vi "MAIN_DSOM.vi"(6 "Y-Max / [V]":dbl=9.0 min=0.0 max=10.0, 7 "X-Max / [V]":dbl=9.0 min=0.0 max=10.0, 8 "Y-Pixels":u32=10 min=2, 9 "Y-Min / [V]":dbl=1.0 min=0.0 max=10.0, 10 "X-Min / [V]":dbl=1.0 min=0.0 max=10.0, 11 "X-Pixels":u32=10 min=2 max=4000) -> ()   [LabVIEW 2009]
uses:
  <vilib>/DAQmx/create/channels.llb/DAQmx Create Channel (DO-Digital Output).vi
  <vilib>/DAQmx/configure/timing.llb/DAQmx Timing (Sample Clock).vi
  <vilib>/DAQmx/write.llb/DAQmx Write (Analog 2D DBL NChan NSamp).vi
  <vilib>/DAQmx/write.llb/DAQmx Write (Digital 1D U8 1Chan NSamp).vi
  Program Files/National Instruments/LabVIEW 2009/resource/objmgr/daqmx.rc
  <vilib>/DAQmx/create/channels.llb/DAQmx Create Channel (AO-Voltage-Basic).vi
  atmcd32d.llb/Shutter_mode typedef.ctl
  atmcd32d.llb/Shutter_type typedef.ctl
  atmcd32d.llb/AcquisitionMode_mode typedef.ctl
  atmcd32d.llb/ReadMode_mode typedef.ctl
  atmcd32d.llb/TriggerMode_mode typedef.ctl
  <vilib>/DAQmx/create/channels.llb/DAQmx Create Channel (CO-Pulse Generation-Frequency).vi
  <vilib>/DAQmx/configure/timing.llb/DAQmx Timing (Implicit).vi
  atmcd32d.llb/EMGainMode_mode typedef.ctl
panel:
  in  "Average or max.\nIntensity":bool
  in  "Scanner Divider":i32=2
  in  "Learning loop":bool=TRUE
  in  "Normalize\nPicture Image":bool=TRUE
  in  "SCANNER EMERGENCY":bool
  out "Cursor Y":i16
  out "Cursor X":i16
  out "Waveform Chart 2":dbl(graph)
  in  "Measurement Mode":enum32{"Picture", "Line", "Point"}(tab)
  out "?":bool
  out "Slide":i32
  out "Programming scanner":u8(slide) caption="Accquire Picture" scale=0.0..100.0
  in  "?":enum32{"Picture", "ROI", "3D-Stack"}(tab)
  in  "Overview":bool
  out "?":bool
  in  "Square":bool
  in  "x-Pixel":u16=100
  in  "y-Pixel":u16=100
  in  "Picture size":dbl=20.0 min=0.1 max=200.0 format="%1.1f um"
  in  "?":dbl=20.0 min=0.1 max=200.0 format="%1.1f um"
  in  "z-Position":dbl=50.0 min=0.0 max=200.0 format="%1.3f um"
  in  "y-Position":dbl=50.0 min=0.0 max=200.0 format="%1.3f um"
  in  "x-Position":dbl=50.0 min=0.0 max=200.0 format="%1.3f um"
  in  "Accquire":bool
  out "?":bool
  in  "lower limit":i32=10 min=0
  in  "x-Pixel":i32=10 min=0
  in  "Square":bool
  in  "y-Pixel":i32=10 min=0
  in  "ROI":bool
  in  "left limit":i32=10 min=0
  out "?":bool
  in  "Zoom":bool
  out "?":bool
  in  "lower left":bool
  in  "upper right":bool
  in  "Step-width [nm]":i32
  in  "Slides":i32
  in  "Stack?":bool
  out "y":dbl format="%.1f nm"
  out "x":dbl format="%.1f nm"
  in  "?":enum32{"Stage", "Mirror"}(radio)
  in  "?":enum32{"Confocal", "High Res"}(radio)=enum."High Res"
  in  "?":enum32{"x-y", "x-z", "y-z"}(radio)
  out "Measurement time / [s]":u32
  in  "Save":bool
  in  "?":enum32{"Stage", "Mirror"}(radio)
  in  "Start Point":dbl
  in  "?":enum32{"Confocal", "High Res"}(radio)
  out "?":bool
  in  "Accquire":bool
  in  "z-Position":dbl=50.0 min=0.0 max=200.0 format="%1.3f um"
  in  "y-Position":dbl=50.0 min=0.0 max=200.0 format="%1.3f um"
  in  "x-Position":dbl=50.0 min=0.0 max=200.0 format="%1.3f um"
  in  "?":enum32{"Picture", "Int Trace", "Video"}(radio)
  in  "?":enum32{"Stage", "Mirror"}(radio)
  in  "Save":bool
  in  "Num of Pictures":i32=3
  out "?":dbl format="%1.3f um"
  out "?":dbl format="%1.3f um"
  out "Intensity Graph":i32[][](graph)
  out "Wavelength_Percent":i32[](array[numeric])
  out "Picture Time":dbl
  out "Exposure Time":u32[][](array[numeric])
  out "Power settings":dbl[][](array[numeric])
  out "Pulse per Wavelength":u8[](array[numeric])
  out "Wavelength":i32[](array[numeric])
  in  "?":T1(tab)=enum."Andor IXon 860"
  in  "Measurement Type":enum32{"Point", "Line", "Area", "Cube"}(ring)
  out "?":bool
  in  "Seed Laser Power 2":i8(knob) min=0 max=100 scale=0.0..100.0
  in  "Laser 2":bool caption="Seed Laser"
  out "?":bool
  in  "PicoQuant Laser Head":bool
  out "Time per Pixel / [ms]":dbl format="%#_6f"
  in  "stop":bool
  in  "Start":bool
  out "Total scanning time / [s]":dbl
  out "Running":bool
  in  "Laser Power Type":T2(ring)
  out "Pictures per pixel":u8
  in  "Number of active Koheras lines":i8=1 min=1 max=8
  out "Actual Power Level / [%]":i8(knob) scale=0.0..100.0
  out "active 1":bool
  out "active 8":bool
  out "active 7":bool
  out "active 6":bool
  out "active 5":bool
  out "active 4":bool
  out "active 3":bool
  out "active 2":bool
  in  "?":T2(tab)
  in  "Number of active Koheras lines":i8=1 min=1 max=8
  out "Command":string
  out "Programming AOTF":bool
  in  "Set Manual":bool
  in  "Exposure\nTime / [us]":u32=100 min=1
  in  "Line 1":i32(slide) min=0 max=100 scale=0.0..100.0
  in  "Line 1":i32(slide)=470 min=470 max=730 scale=470.0..730.0
  in  "Line 2":i32(slide)=470 min=470 max=730 scale=470.0..730.0
  in  "Line 3":i32(slide)=470 min=470 max=730 scale=470.0..730.0
  in  "Line 4":i32(slide)=470 min=470 max=730 scale=470.0..730.0
  in  "Line 5":i32(slide)=470 min=470 max=730 scale=470.0..730.0
  in  "Line 6":i32(slide)=470 min=470 max=730 scale=470.0..730.0
  in  "Line 7":i32(slide)=470 min=470 max=730 scale=470.0..730.0
  in  "Line 8":i32(slide)=470 min=470 max=730 scale=470.0..730.0
  in  "Line 2":i32(slide) min=0 max=100 scale=0.0..100.0
  in  "Line 3":i32(slide) min=0 max=100 scale=0.0..100.0
  in  "Line 4":i32(slide) min=0 max=100 scale=0.0..100.0
  in  "Line 5":i32(slide) min=0 max=100 scale=0.0..100.0
  in  "Line 6":i32(slide) min=0 max=100 scale=0.0..100.0
  in  "Line 7":i32(slide) min=0 max=100 scale=0.0..100.0
  in  "Line 8":i32(slide) min=0 max=100 scale=0.0..100.0
  in  "Exposure\nTime / [us]":u32=100 min=1
  in  "Exposure\nTime / [us]":u32=100 min=1
  in  "Exposure\nTime / [us]":u32=100 min=1
  in  "Exposure\nTime / [us]":u32=100 min=1
  in  "Exposure\nTime / [us]":u32=100 min=1
  in  "Exposure\nTime / [us]":u32=100 min=1
  in  "Exposure\nTime / [us]":u32=100 min=1
  in  "Exposure\nTime 9 / [us]":u32=100 min=1
  in  "Exposure Time\n/ [us]":i32[](array[numeric]) min=1 max=1000000
  in  "Exposure Time\n/ [us]":i32[](array[numeric]) min=1 max=1000000
  in  "Exposure Time\n/ [us]":i32[](array[numeric]) min=1 max=1000000
  in  "Exposure Time\n/ [us]":i32[](array[numeric]) min=1 max=1000000
  in  "Exposure Time\n/ [us]":i32[](array[numeric]) min=1 max=1000000
  in  "Exposure Time\n/ [us]":i32[](array[numeric]) min=1 max=1000000
  in  "Exposure Time\n/ [us]":i32[](array[numeric]) min=1 max=1000000
  in  "Exposure Time\n/ [us]":i32[](array[numeric]) min=1 max=1000000
  in  "Used Power\nEntries":u8=1 min=1
  in  "Power":dbl[](array[numeric]) min=0.0 max=100.0
  in  "Used Power\nEntries":u8=1 min=1
  in  "Power":dbl[](array[numeric]) min=0.0 max=100.0
  in  "Used Power\nEntries":u8=1 min=1
  in  "Power":dbl[](array[numeric]) min=0.0 max=100.0
  in  "Used Power\nEntries":u8=1 min=1
  in  "Power":dbl[](array[numeric]) min=0.0 max=100.0
  in  "Used Power\nEntries":u8=1 min=1
  in  "Power":dbl[](array[numeric]) min=0.0 max=100.0
  in  "Used Power\nEntries":u8=1 min=1
  in  "Power":dbl[](array[numeric]) min=0.0 max=100.0
  in  "Used Power\nEntries":u8=1 min=1
  in  "Power":dbl[](array[numeric]) min=0.0 max=100.0
  in  "Used Power\nEntries":u8=1 min=1
  in  "Line 1":i32(slide)=470 min=470 max=730 scale=470.0..730.0
  in  "Line 2":i32(slide)=470 min=470 max=730 scale=470.0..730.0
  in  "Line 3":i32(slide)=470 min=470 max=730 scale=470.0..730.0
  in  "Line 4":i32(slide)=470 min=470 max=730 scale=470.0..730.0
  in  "Line 5":i32(slide)=470 min=470 max=730 scale=470.0..730.0
  in  "Line 6":i32(slide)=470 min=470 max=730 scale=470.0..730.0
  in  "Line 7":i32(slide)=470 min=470 max=730 scale=470.0..730.0
  in  "Line 8":i32(slide)=470 min=470 max=730 scale=470.0..730.0
  in  "Power":dbl[](array[numeric]) min=0.0 max=100.0
  in  "Proportional\nto Intensity 8":bool caption="Proportional\nto Intensity"
  in  "Exposure\nTime / [us]":u32=100 min=1
  in  "Proportional\nto Intensity 7":bool caption="Proportional\nto Intensity"
  in  "Exposure\nTime / [us]":u32=100 min=1
  in  "Proportional\nto Intensity 6":bool caption="Proportional\nto Intensity"
  in  "Exposure\nTime / [us]":u32=100 min=1
  in  "Proportional\nto Intensity 5":bool caption="Proportional\nto Intensity"
  in  "Exposure\nTime / [us]":u32=100 min=1
  in  "Proportional\nto Intensity 4":bool caption="Proportional\nto Intensity"
  in  "Exposure\nTime / [us]":u32=100 min=1
  in  "Proportional\nto Intensity 3":bool caption="Proportional\nto Intensity"
  in  "Exposure\nTime / [us]":u32=100 min=1
  in  "Proportional\nto Intensity 2":bool caption="Proportional\nto Intensity"
  in  "Exposure\nTime / [us]":u32=100 min=1
  in  "Proportional\nto Intensity":bool
  in  "Steps":u8=2 min=2
  in  "Last Intensity":i8=100 min=0 max=100
  in  "First Intensity":i8=1 min=1 max=100
  in  "Steps":u8=2 min=2
  in  "Last Intensity":i8=100 min=0 max=100
  in  "First Intensity":i8=1 min=1 max=100
  in  "Steps":u8=2 min=2
  in  "Last Intensity":i8=100 min=0 max=100
  in  "First Intensity":i8=1 min=1 max=100
  in  "Steps":u8=2 min=2
  in  "Last Intensity":i8=100 min=0 max=100
  in  "First Intensity":i8=1 min=1 max=100
  in  "Steps":u8=2 min=2
  in  "Last Intensity":i8=100 min=0 max=100
  in  "First Intensity":i8=1 min=1 max=100
  in  "Steps":u8=2 min=2
  in  "Last Intensity":i8=100 min=0 max=100
  in  "First Intensity":i8=1 min=1 max=100
  in  "Steps":u8=2 min=2
  in  "Last Intensity":i8=100 min=0 max=100
  in  "First Intensity":i8=1 min=1 max=100
  in  "Steps":u8=2 min=2
  in  "Last Intensity":i8=100 min=0 max=100
  in  "First Intensity":i8=1 min=1 max=100
  in  "Line 1":i32(slide)=470 min=470 max=730 scale=470.0..730.0
  in  "Line 2":i32(slide)=470 min=470 max=730 scale=470.0..730.0
  in  "Line 3":i32(slide)=470 min=470 max=730 scale=470.0..730.0
  in  "Line 4":i32(slide)=470 min=470 max=730 scale=470.0..730.0
  in  "Line 5":i32(slide)=470 min=470 max=730 scale=470.0..730.0
  in  "Line 6":i32(slide)=470 min=470 max=730 scale=470.0..730.0
  in  "Line 7":i32(slide)=470 min=470 max=730 scale=470.0..730.0
  in  "Line 8":i32(slide)=470 min=470 max=730 scale=470.0..730.0
  in  "Exposure\nTime / [us]":u32=100 min=1
  out "active 9":bool
  out "Interlock":bool
  out "Reset Interlock":bool
  out "?":bool
  in  "Seed Laser Power":i8(knob) min=0 max=100 scale=0.0..100.0
  in  "Laser":bool caption="Seed Laser"
  out "Actual Power Level / [%]":i8(knob) scale=0.0..100.0
  out "Output Photodiode current":i32(graph)
  out "Diode current":cluster{i32, i32, i32}(graph)
  out "Temperature Case":string
  out "Temperature Booster":string
  out "Temperature Preamplifier":string
  out "Temperature Seed Laser":string
  out "SuperK Firmware rev. Hardware":string
  out "SuperK Firmware rev. Display":string
  out "SuperK Firmware rev. Main":string
  out "SuperK Serial No.":string
  out "Board Version":string
  out "Board Serial":string
  out "Board ID":string
  in  "Y-Voltage":dbl=5.0 min=0.0 max=10.0 format="%.6g"
  in  "X-Voltage":dbl=5.0 min=0.0 max=10.0 format="%.6g"
  in  "Set Manual":bool
  in  "Choose Position":dbl min=-10.0 max=10.0 format="%.6g"
  out "Numeric":dbl
  out "Fixed Position / [mm]":dbl format="%.6g"
  in  "Reset Fix Position":bool
  in  "Fix Position":bool
  in  "Move Down":bool
  in  "Move Up":bool
  out "Moving Speed / [%]":i8(knob) scale=0.0..100.0
  in  "Clutch":bool
  out "Actual Microscope Position / [mm]":dbl format="%.6f"
  in  "Numeric 2":i32=10
  out "Differenz":dbl format="%.6f"
  out "actual scan stage position":dbl[](array[numeric]) format="%.6f"
  in  "Shut down\ncamera":bool
  in  "Exposure time / ms":i32=1 min=1 max=5000
  in  "y-pixels":u32=1 min=1 max=1024
  in  "x-pixels":u32=1 min=1 max=1024
  in  "target temperature / [°C]":i32(knob)=40 min=0 max=70 scale=0.0..70.0 scale format="-%.0f"
  out "Temp-stabilized":bool
  out "On/Off":bool
  out "act. temperature / [°C]":dbl
  in  "Cooling":bool
  out "Y-Pixels":dbl
  out "X-Pixels":dbl
  in  "Zoom":bool
  in  "upper right 2":bool
  in  "lower left 2":bool
  in  "x- lower left":u8 max=128
  in  "x- upper right":u8=128 max=128
  in  "y- lower left":u8 max=128
  in  "y-upper right":u8=128 max=128
  in  "gain":i32
  in  "mode":T3
  out "sigx":dbl
  out "sigy":dbl
  out "Signalverlaufsdiagramm":cluster{dbl, dbl}(graph)
  in  "Main Start Clock out":tag="/Dev3/PFI36"
  in  "Analog-Channel Y":tag="Dev1/ao1"
  in  "Analog-Channel X":tag="Dev1/ao0"
  in  "Heidenhain_Seriell":refnum<visa-resource-name>="COM4"
  in  "AOTF Line 1":tag="Dev2/ao0"
  in  "AOTF Line 2":tag="Dev2/ao1"
  in  "AOTF Line 3":tag="Dev2/ao2"
  in  "AOTF Line 4":tag="Dev2/ao3"
  in  "AOTF Line 5":tag="Dev2/ao4"
  in  "AOTF Line 6":tag="Dev2/ao5"
  in  "AOTF Line 7":tag="Dev2/ao6"
  in  "AOTF Line 8":tag="Dev2/ao7"
  in  "Delayed  Main Start Clock in":tag="/Dev3/PFI28"
  in  "AOTF-Digital out":tag="Dev2/port0"
  in  "AOTF-Analog Min Voltage / [V]":dbl
  in  "AOTF-Analog Max Voltage / [V]":dbl=10.0
  in  "Delay / [us]":i32=10 min=1
  in  "Delayed Startclock out":tag="Dev3/ctr1" caption="Delayed Start Clock Out"
  in  "Main Startclock In":tag="/Dev3/PFI0" caption="Main Startclock in"
  in  "20 MHz-Clock":tag="/Dev3/20MHzTimebase" caption="20MHz-Clock for \nDelay-Counting"
  in  "Sample-Clock Out":tag="/Dev1/ao/SampleClock"
  in  "Power Driver":tag="Dev1/port2"
  in  "Clock out":tag="Dev3/ctr7"
  in  "Koheras-AOTF-Controller":refnum<visa-resource-name>="USB0::0x16C7::0x0001::NI-VISA-10001::RAW"
  in  "Koheras Seed Laser":refnum<visa-resource-name>="COM5"
  in  "Picture Clock out":tag="Dev3/ctr3" caption="Pixel Clock out"
  in  "AOTF-Digital switch in":tag="/Dev2/PFI0"
  in  "AOTF-Analog switch in":tag="/Dev2/PFI0"
  in  "Picture Clock Main out":tag="Dev3/ctr5"
  in  "Picture Start Clock in":tag="/Dev3/PFI20"
  in  "Blanking Out":tag="Dev1/port0"
  in  "Picture Clock Main in":tag="/Dev3/PFI12"
  in  "PI E710":u16(ring) items=["COM1", "COM2", "COM3", "COM4", "COM5", "COM6", "COM7", "COM8", "COM9"]
  # "lower left corner"
  # "from cursor"
  # "Pixelsize"
  # "Scan-\ntype"
  # "Laser Power Settings"
  # "Wavelength"
  # "Power"
  # "Koheras-AOTF"
  # "PicoQuant"
  # "Wavelength"
  # "PicoQuant"
  # "Koheras-AOTF"
  # "Wavelength"
  # "In case of proportional exposure to intensity setting, setted exposure time counts for 100% intensity"
  # "PicoQuant"
  # "Koheras-AOTF"
  # "Interlock"
  # "Laser Power Settings"
  # "Temperature"
  # "Koheras\nHardware Version"
  # "Koheras AOTF"
  # "Manual Positioning"
  # "PI  E710-Scanner"
  # "x"
  # "y"
  # "z"
  # "Camera binning"
  # "X"
  # "Camera cooling"
  # "Camera read out"
  # "Scanner"
  # "Timing"
  # "Camera"
  # "AOTF-Analog"
  # "AOTF-Digital"
  # "Mikroskope z-Position"
  # "Position Controller"
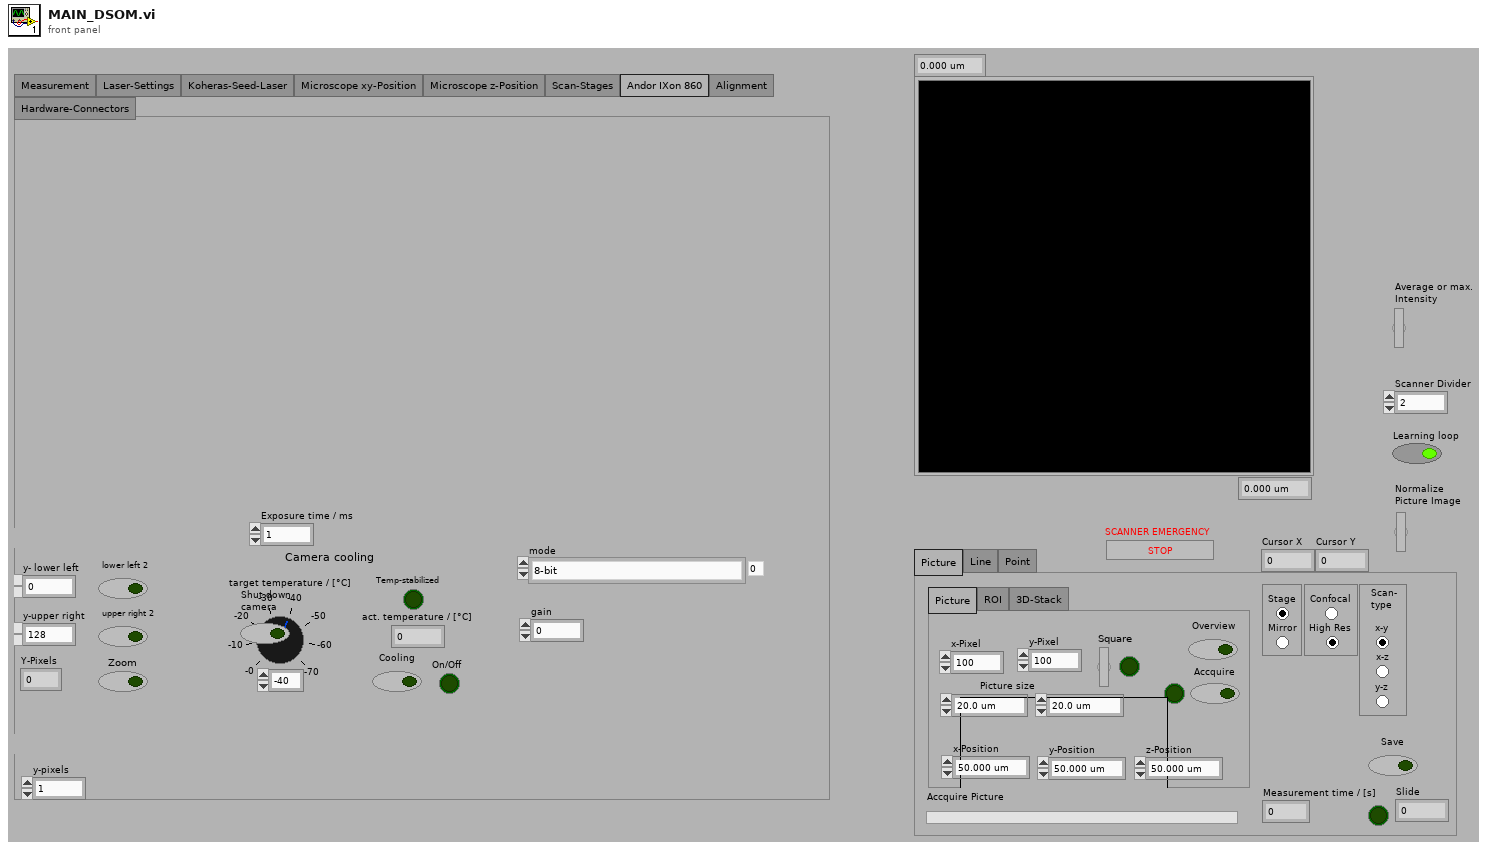
[diagram p1: front panel]
types:
  T1 = enum32{"Measurement", "Laser-Settings", "Koheras-Seed-Laser", "Microscope xy-Position", "Microscope z-Position", "Scan-Stages", "Andor IXon 860", "Alignment", "Hardware-Connectors"}
  T2 = enum32{"Static Power", "Dynamic Power Discrete", "Dynamic Power Ramp"}
  T3 = typedef "EMGainMode_mode typedef.ctl" = enum16{"8-bit", "12-bit", "Linear", "Real"}
  T4 = cluster{string, "cancelled":bool, "error out":errorcluster, bool, "Slides":i32, string}
  T5 = cluster{"Value":i8, "Value":i32[], "Value":i32[], "Set Manual":bool}
  T6 = cluster{"x-Pixel":u16, "y-Pixel":u16, "x-Position":dbl, "y-Position":dbl, "Picture size":dbl, dbl, enum32{"x-y", "x-z", "y-z"}, "z-Position":dbl}
  T7 = typedef "Shutter_mode typedef.ctl" = enum16{"Auto", "Open", "Close"}
  T8 = typedef "Shutter_type typedef.ctl" = enum16{"TTL Low", "TTL High"}
  T9 = typedef "TriggerMode_mode typedef.ctl" = enum16{"Internal", "External", "N/A (2)", "N/A (3)", "N/A (4)", "N/A (5)", "External Start"}
  T10 = typedef "ReadMode_mode typedef.ctl" = enum16{"Full Vertical Binning", "Multi-Track", "Random-Track", "Single-Track", "Image"}
  T11 = typedef "AcquisitionMode_mode typedef.ctl" = enum16{"Reserved (0)", "Single Scan", "Accumulate", "Kinetics", "Fast Kinetics", "Run Till Abort", "Reserved (6)", "Reserved (7)", "Reserved (8)", "Time Delayed Integration"}
  T12 = cluster{"dimension size":i32, "dimension size":i32, "dimension size":i32, "dimension size":i32}
  T13 = cluster{"Acquis. mode":T11, "Read mode":T10, "Horizontal bin":i32, "Vertical bin":i32, "x-min":i32, "x-max":i32, "y-min":i32, "y-max":i32, "Trigger mode":T9, " Exposure time":sgl, "AD channel":i32, "Num of Pictures":i32, "Shutter type":T8, "Shutter mode":T7, "Shutter\nopeningtime":i32, "Shutter\nclosingtime":i32}
  T14 = cluster{cluster{"dimension size":i32, "dimension size":i32, "dimension size":i32, "dimension size":i32}, i32[], "Picture Data":dbl[][], u32[], "millisecond timer value":u32, dbl[][], i32[][], cluster{"Acquis. mode":T11, "Read mode":T10, "Horizontal bin":i32, "Vertical bin":i32, "x-min":i32, "x-max":i32, "y-min":i32, "y-max":i32, "Trigger mode":T9, " Exposure time":sgl, "AD channel":i32, "Num of Pictures":i32, "Shutter type":T8, "Shutter mode":T7, "Shutter\nopeningtime":i32, "Shutter\nclosingtime":i32}, "Boolean array":bool[], cluster{dbl[], dbl[]}, "cluster":cluster{"x-Pixel":u16, "y-Pixel":u16, "x-Position":dbl, "y-Position":dbl, "Picture size":dbl, dbl, enum32{"x-y", "x-z", "y-z"}, "z-Position":dbl}}
  T15 = cluster{"Boolean array[0]":bool, "Boolean array[1]":bool, "Boolean array[2]":bool, "Boolean array[3]":bool, "Boolean array[4]":bool, "Boolean array[5]":bool, "Boolean array[6]":bool, "Boolean array[7]":bool, "Boolean array[8]":bool}
  T16 = cluster{dbl, "X-Pixels":u32, "Y-Pixels":u32, "X-Min / [V]":dbl, "X-Max / [V]":dbl, "Y-Min / [V]":dbl, "Y-Max / [V]":dbl}
  T17 = cluster{"AOTF Line 1":tag, "AOTF Line 2":tag, "AOTF Line 3":tag, "AOTF Line 4":tag, "AOTF Line 5":tag, "AOTF Line 6":tag, "AOTF Line 7":tag, "AOTF Line 8":tag}
  T18 = cluster{"Main Start Clock out":tag, "Analog-Channel X":tag, "Analog-Channel Y":tag, "Sample-Clock Out":tag}
  T19 = cluster{"AOTF-Digital switch in":tag, "Picture Clock out":tag, "AOTF-Analog switch in":tag, "Picture Clock Main out":tag, "Picture Start Clock in":tag, "Picture Clock Main in":tag, "Blanking Out":tag, "Delayed  Main Start Clock in":tag, "AOTF-Digital out":tag}
  T20 = cluster{"Delay / [us]":i32, "Delayed Startclock out":tag, "Main Startclock In":tag, "20 MHz-Clock":tag}
  T21 = cluster{"Value":bool, "Value":bool[], "Value":bool[], "Set Manual":bool}
  T22 = cluster{"Cursor.Cursor X":dbl, "Cursor.Cursor Y":dbl}
  T23 = cluster{"x- lower left":u8, "y- lower left":u8, "x- upper right":u8, "y-upper right":u8}
  T24 = cluster{cluster{"x- lower left":u8, "y- lower left":u8, "x- upper right":u8, "y-upper right":u8}, cluster{"dimension size":i32, "dimension size":i32, "dimension size":i32, "dimension size":i32}, "lower left 2":bool, "upper right 2":bool}
  T25 = cluster{"left limit":i32, "lower limit":i32, "x-Pixel":i32, "y-Pixel":i32}
  T26 = cluster{"left limit":i32, i32, "lower limit":i32, i32}
  T27 = typedef "Error Code Enum typedef.ctl" = enum32{"N/A (0)", "DRV_ERROR_CODES", "DRV_SUCCESS", "DRV_VXDNOTINSTALLED", "DRV_ERROR_SCAN", "DRV_ERROR_CHECK_SUM", "DRV_ERROR_FILELOAD", "DRV_UNKNOWN_FUNC", "DRV_ERROR_VXD_INIT", "DRV_ERROR_ADDRESS", "DRV_ERROR_PAGELOCK", "DRV_ERROR_PAGEUNLOCK", "DRV_ERROR_BOARDTEST", "DRV_ERROR_ACK", "DRV_ERROR_UP_FIFO", "DRV_ERROR_PATTERN", "N/A (16)", "DRV_ACQUISITION_ERRORS", "DRV_ACQ_BUFFER", "DRV_ACQ_DOWNFIFO_FULL", "DRV_PROC_UNKONWN_INSTRUCTION", "DRV_ILLEGAL_OP_CODE", "DRV_KINETIC_TIME_NOT_MET", "DRV_ACCUM_TIME_NOT_MET", "DRV_NO_NEW_DATA", "N/A (25)", "DRV_SPOOLERROR", "N/A (27)", "N/A (28)", "N/A (29)", "N/A (30)", "N/A (31)", "N/A (32)", "DRV_TEMPERATURE_CODES", "DRV_TEMPERATURE_OFF", "DRV_TEMPERATURE_NOT_STABILIZED", "DRV_TEMPERATURE_STABILIZED", "DRV_TEMPERATURE_NOT_REACHED", "DRV_TEMPERATURE_OUT_RANGE", "DRV_TEMPERATURE_NOT_SUPPORTED", "DRV_TEMPERATURE_DRIFT", "N/A (41)", "N/A (42)", "N/A (43)", "N/A (44)", "N/A (45)", "N/A (46)", "N/A (47)", "N/A (48)", "DRV_GENERAL_ERRORS", "DRV_INVALID_AUX", "DRV_COF_NOTLOADED", "DRV_FPGAPROG", "DRV_FLEXERROR", "DRV_GPIBERROR", "N/A (55)", "N/A (56)", "N/A (57)", "N/A (58)", "N/A (59)", "N/A (60)", "N/A (61)", "N/A (62)", "N/A (63)", "DRV_DATATYPE", "DRV_DRIVER_ERRORS", "DRV_P1INVALID", "DRV_P2INVALID", "DRV_P3INVALID", "DRV_P4INVALID", "DRV_INIERROR", "DRV_COFERROR", "DRV_ACQUIRING", "DRV_IDLE", "DRV_TEMPCYCLE", "DRV_NOT_INITIALIZED", "DRV_P5INVALID", "DRV_P6INVALID", "DRV_INVALID_MODE", "DRV_INVALID_FILTER", "DRV_I2CERRORS", "DRV_I2CDEVNOTFOUND", "DRV_I2CTIMEOUT", "DRV_P7INVALID", "N/A (84)", "N/A (85)", "N/A (86)", "N/A (87)", "N/A (88)", "N/A (89)", "DRV_IOCERROR", "DRV_VRMVERSIONERROR"}
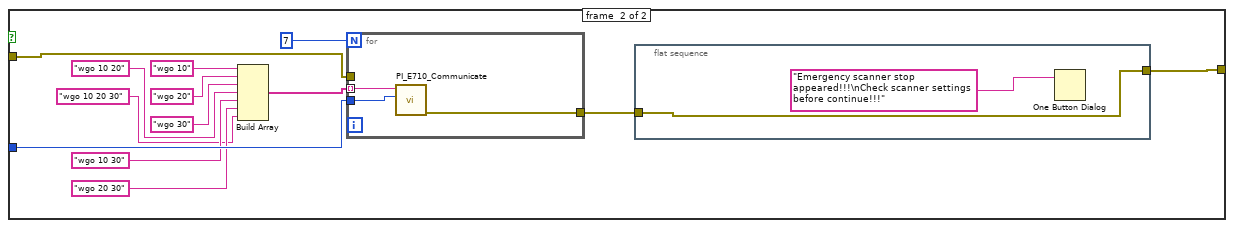
[diagram p2: hidden frame]
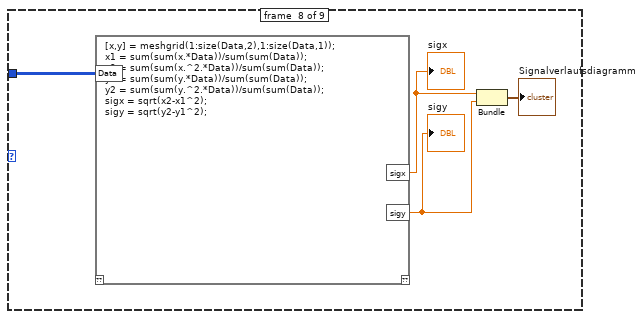
[diagram p9: hidden frame]
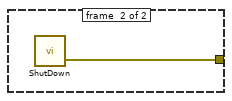
[diagram p11: hidden frame]
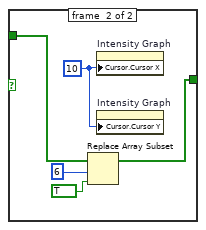
[diagram p12: hidden frame]
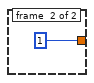
[diagram p13: hidden frame]
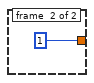
[diagram p14: hidden frame]
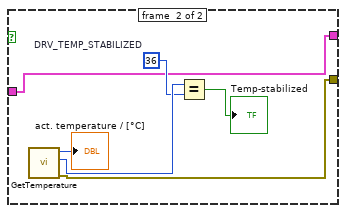
[diagram p15: hidden frame]
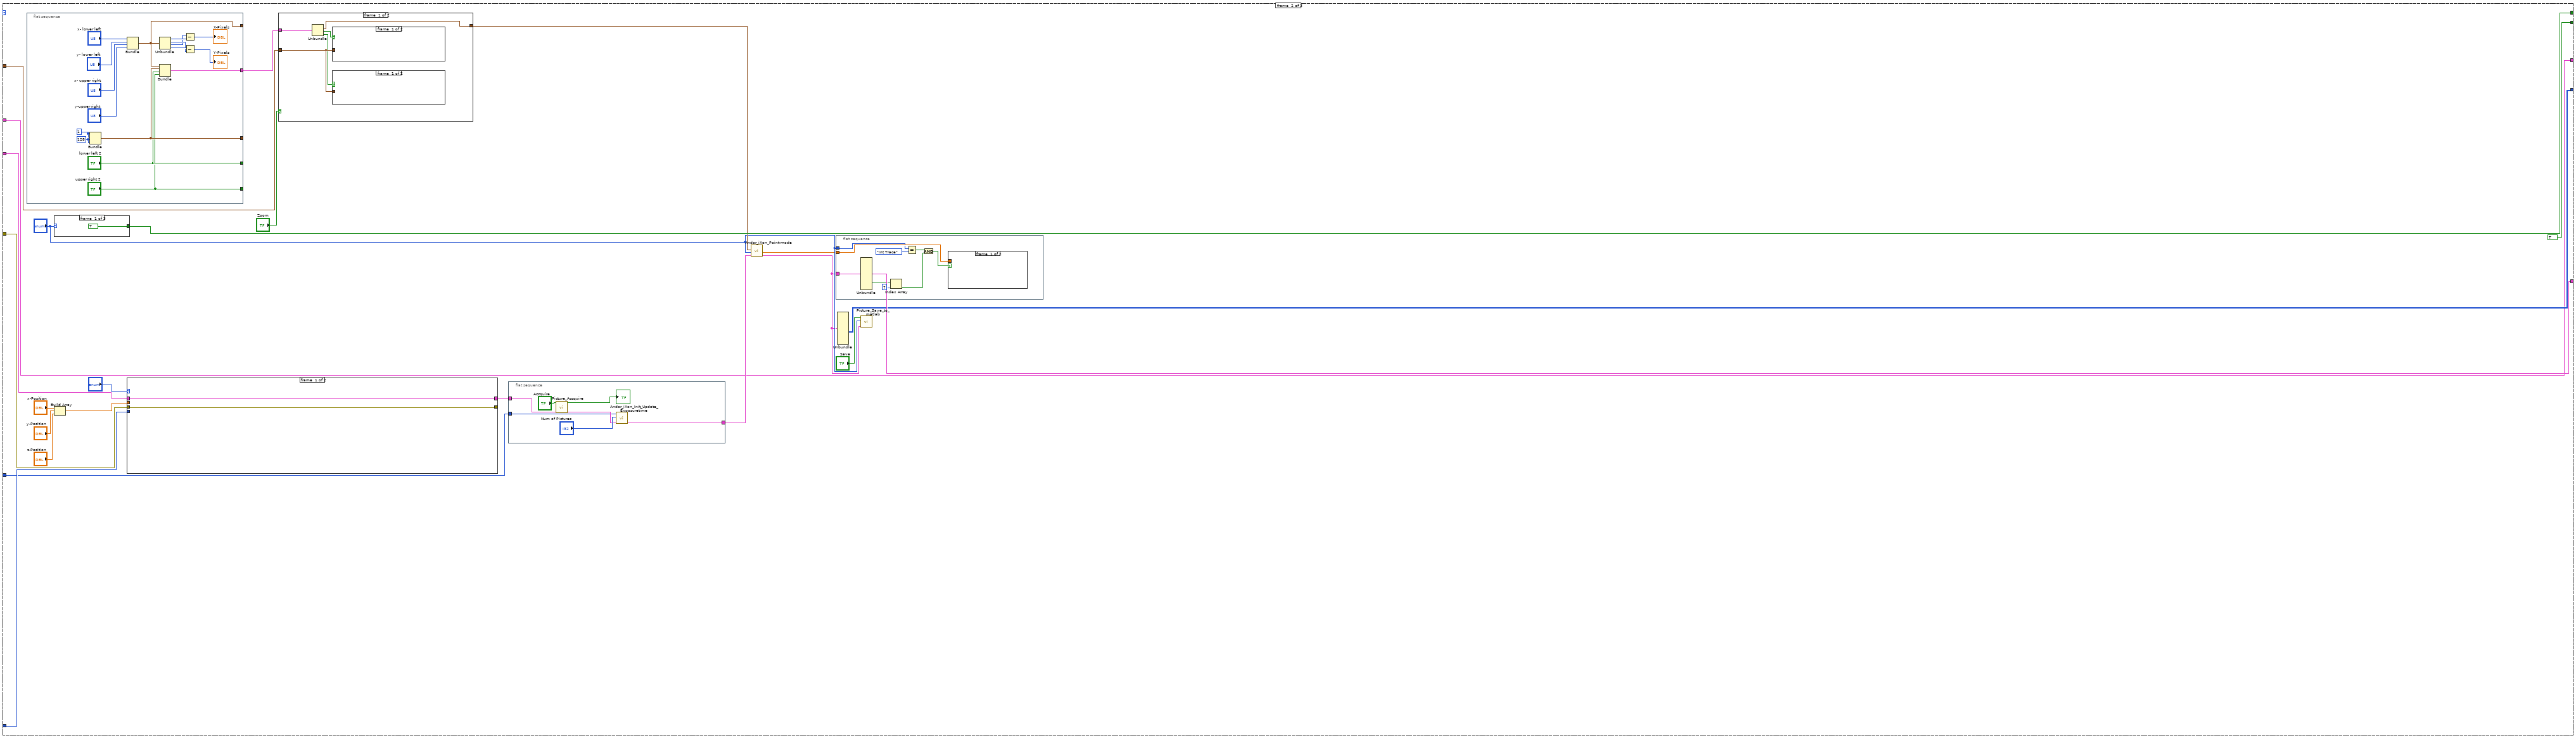
[diagram p17: hidden frame]
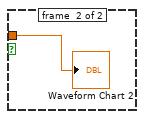
[diagram p18: hidden frame]
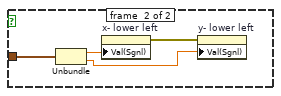
[diagram p19: hidden frame]
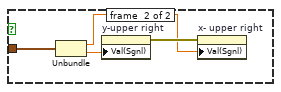
[diagram p20: hidden frame]
diagram:
  w3 = 1  # System no.
  w18 = 10214 items=["High"=10192, "Low"=10214] ("Idle State 2")
  w8 = bool[] [FALSE, FALSE, FALSE, FALSE, FALSE, FALSE, FALSE, FALSE] ("appended array")
  w19 = 10123 items=["Finite Samples"=10178, "Continuous Samples"=10123] ("sample mode")
  w28 = 1 items=["one channel for each line", "one channel for all lines"] ("line grouping")
  n1 = flat-sequence {
    tunnel: [w72] -> w2
    frame #0 {
      w48 = 0.0 ("element")
      w60 = 3  # Num of Pictures
      w51 = 128  # y-max
      w52 = 128  # y-min
      w53 = 1  # x-max
      w54 = 1  # x-min
      w64 = 1  # Vertical bin
      w65 = 1  # Horizontal bin
      w56 = 0  # Shutter closingtime
      w57 = 0  # Shutter openingtime
      w58 = Shutter_mode_typedef."Auto"  # Shutter mode
      w59 = Shutter_type_typedef."TTL Low"  # Shutter type
      w61 = 0  # AD channel
      w62 = sgl 0.05  # Exposure time
      w63 = TriggerMode_mode_typedef."Internal"  # Trigger mode
      w66 = ReadMode_mode_typedef."Image"  # Read mode
      w67 = AcquisitionMode_mode_typedef."Kinetics"  # Acquis. mode
      w76 = 128 ("dimension size")
      w77 = 1 ("dimension size")
      w73 = dbl[][] []  # Picture Data
      w91 = 1  # element
      n2 = Build Array "Scanner 1 Range"(0.0 ("y"), 200.0 ("y")) -> (w83:dbl[])
      n3 = Build Array "Scanner 2 Range"(0.0 ("y"), 200.0 ("y")) -> (w82:dbl[])
      n4 = Build Array "Scanner 3 Range"(0.0 ("element"), 200.0 ("y")) -> (w81:dbl[])
      n5 = Initialize Array "Pixels_Confocal"(w91, 512 ("dimension size"), 512 ("dimension size")) -> (w68:i32[][])
      n6 = Build Array "Scanner position"(w48, w48, w48) -> (w46:dbl[])
      n7 = Bundle("dimension size"=w77, "dimension size"=w77, "dimension size"=w76, "dimension size"=w76) -> (w75:T12)  [unwired: 1 out]
      n8 = Initialize Array(0, 16384 ("dimension size")) -> (w74:i32[])
      n9 = Build Array "Scanner range"(w83, w82, w81) -> (w69:dbl[][])
      n10 = Bundle "Camera config"("Acquis. mode"=w67, "Read mode"=w66, "Horizontal bin"=w65, "Vertical bin"=w64, "x-min"=w54, "x-max"=w53, "y-min"=w52, "y-max"=w51, "Trigger mode"=w63, "Exposure time"=w62, "AD channel"=w61, "Num of Pictures"=w60, "Shutter type"=w59, "Shutter mode"=w58, "Shutter\nopeningtime"=w57, "Shutter\nclosingtime"=w56) -> (w55:T13)  [unwired: 1 out]
      n11 = Bundle "Scanner pos"(w46, w46) -> (w47:cluster{dbl[], dbl[]})  [unwired: 1 out]
      n12 = Tick Count (ms)() -> (millisecond timer value=w70:u32)
      n13 = Number To Boolean Array(number=u32 0) -> (Boolean array=w49:bool[])
      n14 = Bundle(w75, w74, "Picture Data"=w73, u32[] [], "millisecond timer value"=w70, w69, w68, w55, "Boolean array"=w49, w47, "cluster"=T6 {"x-Pixel"=0, "y-Pixel"=0, "x-Position"=0.0, "y-Position"=0.0, "Picture size"=0.0, 0.0, enum."x-y", "z-Position"=0.0}) -> (w72:T14)  [unwired: 1 out]
    }
  }
  n15 = while {
    stop <- w96 stop-if-true
    # "AOTF-Preparation Task"
    n16 = Wait Until Next ms Multiple(millisecond multiple=u32 100) -> ()  [unwired: 1 out]
    n17 = property on="Running" class="Bool (strict)"() -> ("Value"=w94:bool)  [unwired: 2 in, 2 out]
    n18 = case shown="False" w94 {
      tunnel: "AOTF-Analog Min Voltage / [V]" -> [w106 _]
      tunnel: "AOTF-Analog Max Voltage / [V]" -> [w105 _]
      frame #0 {
        n19 = Scale By Power Of 2(n="Number of active Koheras lines", x=1.0) -> (x*2^n=w113:dbl)
        n20 = Decrement(x=w113) -> (x-1=w112:dbl)
        n21 = case shown="\"Static Power\", Default" "?" {
          tunnel: "Number of active Koheras lines" -> [w129 w173 w264]
          tunnel: [w142 w188 w318] -> w109
          tunnel: [w129 w189 w319] -> w108
          tunnel: [w144 w174 w266] -> w107
          tunnel: [w138 w186 w260] -> w104
          tunnel: w106 -> [w140 w184 w258]
          tunnel: w105 -> [w141 w185 w259]
          tunnel: [w126 w172 w257] -> w98
          tunnel: [w125 i32[] [] i32[] []] -> w97
          frame #0 {
            n22 = Build Array "Power"("Line 1", "Line 2", "Line 3", "Line 4", "Line 5", "Line 6", "Line 7", "Line 8") -> (w125:i32[])
            n23 = for {
              N: 8 -> [_]
              tunnel: w141 -> [w166]
              tunnel: w140 -> [w165]
              tunnel: w125 -> [w164] mode=indexing
              tunnel: [w162] -> w138 mode=indexing
              n24 = Subtract(x=w166, y=w165) -> (x-y=w167:dbl)
              n25 = Divide(x=w164, y=i8 100) -> (x/y=w169:dbl)
              n26 = Multiply(x=w167, y=w169) -> (x*y=w168:dbl)
              n27 = Add(x=w165, y=w168) -> (x+y=w163:dbl)
              n28 = Build Array(w163) -> (w162:dbl[])
            }
            n29 = Build Array "Power"("Exposure\nTime / [us]", "Exposure\nTime / [us]", "Exposure\nTime / [us]", "Exposure\nTime / [us]", "Exposure\nTime / [us]", "Exposure\nTime / [us]", "Exposure\nTime / [us]", "Exposure\nTime / [us]") -> (w127:u32[])
            n30 = Build Array "Wavelength"("Line 1", "Line 2", "Line 3", "Line 4", "Line 5", "Line 6", "Line 7", "Line 8") -> (w142:i32[])
            n31 = Build Array(w127) -> (w128:u32[][])
            n32 = Transpose 2D Array(2D array=w128) -> (transposed array=w126:u32[][])
            n33 = Initialize Array(1 ("dimension size"), 8 ("dimension size")) -> (w144:i32[])
          }
          frame #1 {
            n34 = Array Subset(array="Power", index=0, length="Used Power\nEntries") -> (w207:dbl[])
            n35 = Array Subset(array="Power", index=0, length="Used Power\nEntries") -> (w206:dbl[])
            n36 = Array Subset(array="Power", index=0, length="Used Power\nEntries") -> (w220:dbl[])
            n37 = Array Subset(array="Power", index=0, length="Used Power\nEntries") -> (w209:dbl[])
            n38 = Array Subset(array="Power", index=0, length="Used Power\nEntries") -> (w208:dbl[])
            n39 = Array Subset(array="Power", index=0, length="Used Power\nEntries") -> (w205:dbl[])
            n40 = Array Subset(array="Power", index=0, length="Used Power\nEntries") -> (w202:dbl[])
            n41 = Array Subset(array="Power", index=0, length="Used Power\nEntries") -> (w199:dbl[])
            n42 = Build Array "Power"(w220, w209, w208, w207, w206, w205, w202, w199) -> (w187:dbl[][])
            n43 = for {
              N: 8 -> [_]
              tunnel: w187 -> [w234] mode=indexing
              tunnel: [w233] -> w186 mode=indexing
              tunnel: w185 -> [w232]
              tunnel: w184 -> [w231]
              n44 = Array Size(array=w234) -> (size(s)=w235:i32)
              n45 = for {
                N: w235 -> [_]
                tunnel: w234 -> [w238] mode=indexing
                tunnel: [w239] -> w233 mode=indexing
                tunnel: w232 -> [w237]
                tunnel: w231 -> [w236]
                n46 = Subtract(x=w237, y=w236) -> (x-y=w240:dbl)
                n47 = Divide(x=w238, y=i8 100) -> (x/y=w242:dbl)
                n48 = Multiply(x=w240, y=w242) -> (x*y=w241:dbl)
                n49 = Add(x=w236, y=w241) -> (x+y=w239:dbl)
              }
            }
            n50 = Build Array("Used Power\nEntries", "Used Power\nEntries", "Used Power\nEntries", "Used Power\nEntries", "Used Power\nEntries", "Used Power\nEntries", "Used Power\nEntries", "Used Power\nEntries") -> (w174:u8[])
            n51 = for {
              N: w173 -> [_]
              tunnel: w174 -> [w246] mode=indexing
              shift-right: [w245] -> w189
              shift-left: u8 0 -> [w244]
              n52 = Add(x=w246, y=w244) -> (x+y=w245:u8)
            }
            n53 = Build Array "Wavelength"("Line 1", "Line 2", "Line 3", "Line 4", "Line 5", "Line 6", "Line 7", "Line 8") -> (w188:i32[])
            n54 = Build Array("Exposure Time\n/ [us]", "Exposure Time\n/ [us]", "Exposure Time\n/ [us]", "Exposure Time\n/ [us]", "Exposure Time\n/ [us]", "Exposure Time\n/ [us]", "Exposure Time\n/ [us]", "Exposure Time\n/ [us]") -> (w172:i32[][])
          }
          frame #2 {
            n55 = Build Array("Steps", "Steps", "Steps", "Steps", "Steps", "Steps", "Steps", "Steps") -> (w266:u8[])
            n56 = call "Laser-Power-Loop.vi"("Steps"="Steps", "AOTF-Analog Max Voltage"=w259, "AOTF-Analog Min Voltage"=w258, "Last Intensity"="Last Intensity", "First Intensity"="First Intensity") -> ("Power"=w252:dbl[], "Power-Absolute"=w298:dbl[])  [unwired: 5 out]
            n57 = call "Laser-Power-Loop.vi"("Steps"="Steps", "AOTF-Analog Max Voltage"=w259, "AOTF-Analog Min Voltage"=w258, "Last Intensity"="Last Intensity", "First Intensity"="First Intensity") -> ("Power"=w251:dbl[], "Power-Absolute"=w294:dbl[])  [unwired: 5 out]
            n58 = call "Laser-Power-Loop.vi"("Steps"="Steps", "AOTF-Analog Max Voltage"=w259, "AOTF-Analog Min Voltage"=w258, "Last Intensity"="Last Intensity", "First Intensity"="First Intensity") -> ("Power"=w250:dbl[], "Power-Absolute"=w290:dbl[])  [unwired: 5 out]
            n59 = call "Laser-Power-Loop.vi"("Steps"="Steps", "AOTF-Analog Max Voltage"=w259, "AOTF-Analog Min Voltage"=w258, "Last Intensity"="Last Intensity", "First Intensity"="First Intensity") -> ("Power"=w249:dbl[], "Power-Absolute"=w286:dbl[])  [unwired: 5 out]
            n60 = call "Laser-Power-Loop.vi"("Steps"="Steps", "AOTF-Analog Max Voltage"=w259, "AOTF-Analog Min Voltage"=w258, "Last Intensity"="Last Intensity", "First Intensity"="First Intensity") -> ("Power"=w256:dbl[], "Power-Absolute"=w314:dbl[])  [unwired: 5 out]
            n61 = call "Laser-Power-Loop.vi"("Steps"="Steps", "AOTF-Analog Max Voltage"=w259, "AOTF-Analog Min Voltage"=w258, "Last Intensity"="Last Intensity", "First Intensity"="First Intensity") -> ("Power"=w255:dbl[], "Power-Absolute"=w310:dbl[])  [unwired: 5 out]
            n62 = call "Laser-Power-Loop.vi"("Steps"="Steps", "AOTF-Analog Max Voltage"=w259, "AOTF-Analog Min Voltage"=w258, "Last Intensity"="Last Intensity", "First Intensity"="First Intensity") -> ("Power"=w254:dbl[], "Power-Absolute"=w306:dbl[])  [unwired: 5 out]
            n63 = call "Laser-Power-Loop.vi"("Steps"="Steps", "AOTF-Analog Max Voltage"=w259, "AOTF-Analog Min Voltage"=w258, "Last Intensity"="Last Intensity", "First Intensity"="First Intensity") -> ("Power"=w253:dbl[], "Power-Absolute"=w302:dbl[])  [unwired: 5 out]
            n64 = Array Subset(array=w266, index=0, length=w264) -> (w263:u8[])
            n65 = Array Max & Min(array=w263) -> (max value=w262:u8)  [unwired: 3 out]
            n66 = Build Array "Power"(w314, w310, w306, w302, w298, w294, w290, w286) -> (w260:dbl[][])
            n67 = Build Array "Power"(w256, w255, w254, w253, w252, w251, w250, w249) -> (w248:dbl[][])
            n68 = Build Array("Proportional\nto Intensity", "Proportional\nto Intensity 2", "Proportional\nto Intensity 3", "Proportional\nto Intensity 4", "Proportional\nto Intensity 5", "Proportional\nto Intensity 6", "Proportional\nto Intensity 7", "Proportional\nto Intensity 8") -> (w268:bool[])
            n69 = Build Array("Exposure\nTime / [us]", "Exposure\nTime / [us]", "Exposure\nTime / [us]", "Exposure\nTime / [us]", "Exposure\nTime / [us]", "Exposure\nTime / [us]", "Exposure\nTime / [us]", "Exposure\nTime / [us]") -> (w269:u32[])
            n70 = Initialize Array(0 ("element"), w264, w262) -> (w261:i32[][])
            n71 = for {
              N: w264 -> [_]
              tunnel: w266 -> [w335] mode=indexing
              tunnel: w269 -> [w334] mode=indexing
              tunnel: w268 -> [w333] mode=indexing
              tunnel: [w332] -> w257 mode=indexing
              tunnel: w261 -> [w331] mode=indexing
              tunnel: w248 -> [w329] mode=indexing
              n72 = Reverse 1D Array(array=w329) -> (reversed array=w330:dbl[])
              n73 = case shown="True" w333 {
                tunnel: w335 -> [w339 w348]
                tunnel: w334 -> [w338 w347]
                tunnel: [w337 w345] -> w332
                tunnel: w331 -> [w336 w346]
                tunnel: w330 -> [_ w344]
                frame #0 {
                  n74 = for {
                    N: w339 -> [_]
                    tunnel: w338 -> [w341]
                    shift-right: [w342] -> w337
                    shift-left: w336 -> [w343]
                    i -> [w340]
                    n75 = Replace Array Subset(array=w343, new element=w341, index=w340) -> (w342:i32[])
                  }
                }
                frame #1 {
                  n76 = for {
                    N: w348 -> [_]
                    tunnel: w347 -> [w351]
                    shift-right: [w355] -> w345
                    shift-left: w346 -> [w356]
                    tunnel: w344 -> [w350] mode=indexing
                    i -> [w354]
                    n77 = Reciprocal(x=w350) -> (1/x=w349:dbl)
                    n78 = Multiply(x=w351, y=w349) -> (x*y=w352:dbl)
                    n79 = To Long Integer(number=w352) -> (32bit integer=w353:i32)
                    n80 = Replace Array Subset(array=w356, new element=w353, index=w354) -> (w355:i32[])
                  }
                }
              }
            }
            n81 = for {
              N: w264 -> [_]
              tunnel: w266 -> [w359] mode=indexing
              shift-right: [w358] -> w319
              shift-left: u8 0 -> [w357]
              n82 = Add(x=w359, y=w357) -> (x+y=w358:u8)
            }
            n83 = Build Array "Wavelength"("Line 1", "Line 2", "Line 3", "Line 4", "Line 5", "Line 6", "Line 7", "Line 8") -> (w318:i32[])
          }
        }
        "Wavelength" <- w109
        "Pictures per pixel" <- w108
        "Pulse per Wavelength" <- w107
        "Power settings" <- w104
        "Exposure Time" <- w98
        "Wavelength_Percent" <- w97
        n84 = Number To Boolean Array(number=w112) -> (Boolean array=w123:bool[])
        n85 = Array To Cluster(array=w123) -> (cluster=w122:T15)
        n86 = Unbundle(w122) -> ("Boolean array[0]"=→"active 1":bool, "Boolean array[1]"=→"active 2":bool, "Boolean array[2]"=→"active 3":bool, "Boolean array[3]"=→"active 4":bool, "Boolean array[4]"=→"active 5":bool, "Boolean array[5]"=→"active 6":bool, "Boolean array[6]"=→"active 7":bool, "Boolean array[7]"=→"active 8":bool)  [unwired: 1 out]
        n87 = Array Max & Min(array=w98) -> (max value=w103:u32)  [unwired: 3 out]
        n88 = Divide(x=w103, y=0.9) -> (x/y=w101:dbl)
        n89 = Divide(x=w101, y=1000.0) -> (x/y=→"Picture Time":dbl)
      }
      frame #1 {
      }
    }
    n90 = property on="active 9" class="Bool (strict)" props=["Value"]() -> ()  [unwired: 2 in, 3 out]
    n91 = property on="stop" class="Bool (strict)"() -> ("Value"=w96:bool)  [unwired: 2 in, 2 out]
  }
  n92 = property on="stop" class="Bool (strict)"("Val(Sgnl)"=FALSE ("Value (Signaling)")) -> ()  [unwired: 2 in, 2 out]
  n93 = while {
    shift-right: [w396] -> _
    shift-left: 0 -> [w390]
    shift-right: [w383] -> _
    shift-left: FALSE -> [w385]
    shift-right: [w381] -> _
    shift-left: i8 0 ("Seed Laser Power") -> [w380]
    shift-right: [w378] -> _
    shift-left: 0 -> [w377]
    shift-right: [w375] -> _
    shift-left: T5 {"Value"=0, "Value"=[], "Value"=[], "Set Manual"=FALSE} -> [w374]
    stop <- w437 stop-if-true
    # "Main Measurement Task"
    n94 = Wait Until Next ms Multiple(millisecond multiple=u32 100) -> ()  [unwired: 1 out]
    n95 = case shown="\"Koheras-Seed-Laser\"" "?" {
      tunnel: "Laser" -> [_ _ w561 _ _ _ _]
      tunnel: "Laser 2" -> [w558 _ _ _ _ _ _]
      tunnel: "Seed Laser Power 2" -> [w557 _ _ _ _ _ _]
      tunnel: "Seed Laser Power" -> [_ _ w562 _ _ _ _]
      tunnel: [w558 w560 w561 w563 w566 w568 w570] -> w383
      tunnel: [w557 w559 w562 w564 w565 w567 w569] -> w381
      tunnel: w385 -> [_ w560 _ w563 w566 w568 w570]
      tunnel: w380 -> [_ w559 _ w564 w565 w567 w569]
      frame #0 {
      }
      frame #1 {
      }
      frame #2 {
      }
      frame #3 {
      }
      frame #4 {
      }
      frame #5 {
      }
      frame #6 {
      }
    }
    n96 = property on="Picture Time" class="DigNum (strict)"() -> ("Value"=w408:dbl)  [unwired: 2 in, 2 out]
    n97 = property on="Pictures per pixel" class="DigNum (strict)"() -> ("Value"=w414:u8)  [unwired: 2 in, 2 out]
    n98 = Divide(x=w408, y=1000) -> (x/y=w417:dbl)
    n99 = Increment(x=w414) -> (x+1=w405:u8)
    n100 = call "Koheras_Laser_switch.vi"("Koheras Seed Laser"=w383, "Change-Detector in"=w385, "Modus in"=w390) -> ("Answer Length Out"=w391:i32[], "Command Out"=w392:string[], "Modus Out"=w389:i32)  [unwired: 6 out]
    n101 = Reciprocal(x=w417) -> (1/x=w409:dbl)
    n102 = Multiply(x=w405, y=0.9) -> (x*y=w406:dbl)
    n103 = Divide(x=w405, y=w406) -> (x/y=w407:dbl)
    n104 = Increment(x="X-Pixels") -> (x+1=w442:u32)
    n105 = Divide(x=w409, y=w405) -> (x/y=w415:dbl)
    n106 = Increment(x="Y-Pixels") -> (x+1=w439:u32)
    n107 = Multiply(x=w442, y=w439) -> (x*y=w441:u32)
    n108 = Multiply(x=w415, y=w407) -> (x*y=w416:dbl)
    n109 = Reciprocal(x=w415) -> (1/x=w436:dbl)
    n110 = call "Koheras_Seed_Laser_Power.vi"("New Power"=w381, "Answer Length In"=w391, "Command In"=w392, "Setted Seed Laser Power"=w380, "Modus In"=w389) -> ("Answer Length Out"=w393:i32[], "Command Out"=w394:string[], "Modus Out"=w395:i32)  [unwired: 1 in, 3 out]
    n111 = Multiply(x=w439, y=0.003) -> (x*y=w445:dbl)
    n112 = Multiply(x=w436, y=w441) -> (x*y=w440:dbl)
    n113 = Bundle "Pixel-Configuration"(w416, "X-Pixels"="X-Pixels", "Y-Pixels"="Y-Pixels", "X-Min / [V]"="X-Min / [V]", "X-Max / [V]"="X-Max / [V]", "Y-Min / [V]"="Y-Min / [V]", "Y-Max / [V]"="Y-Max / [V]") -> (w421:T16)  [unwired: 1 out]
    n114 = Bundle "AOTF-Analog-Lines"("AOTF Line 1"="AOTF Line 1", "AOTF Line 2"="AOTF Line 2", "AOTF Line 3"="AOTF Line 3", "AOTF Line 4"="AOTF Line 4", "AOTF Line 5"="AOTF Line 5", "AOTF Line 6"="AOTF Line 6", "AOTF Line 7"="AOTF Line 7", "AOTF Line 8"="AOTF Line 8") -> (w426:T17)  [unwired: 1 out]
    n115 = Bundle "Scanner-Analog-Lines"("Main Start Clock out"="Main Start Clock out", "Analog-Channel X"="Analog-Channel X", "Analog-Channel Y"="Analog-Channel Y", "Sample-Clock Out"="Sample-Clock Out") -> (w371:T18)  [unwired: 1 out]
    n116 = Multiply(x=1000.0 ("y"), y=w436) -> (x*y=→"Time per Pixel / [ms]":dbl)
    n117 = Add(x=w440, y=w445) -> (x+y=→"Total scanning time / [s]":dbl)
    n118 = Bundle("AOTF-Digital switch in"="AOTF-Digital switch in", "Picture Clock out"="Picture Clock out", "AOTF-Analog switch in"="AOTF-Analog switch in", "Picture Clock Main out"="Picture Clock Main out", "Picture Start Clock in"="Picture Start Clock in", "Picture Clock Main in"="Picture Clock Main in", "Blanking Out"="Blanking Out", "Delayed  Main Start Clock in"="Delayed  Main Start Clock in", "AOTF-Digital out"="AOTF-Digital out") -> (w368:T19)  [unwired: 1 out]
    n119 = Bundle("Delay / [us]"="Delay / [us]", "Delayed Startclock out"="Delayed Startclock out", "Main Startclock In"="Main Startclock In", "20 MHz-Clock"="20 MHz-Clock") -> (w399:T20)  [unwired: 1 out]
    n120 = property on="Wavelength_Percent" class="Arr (strict)"() -> ("Value"=w373:i32[])  [unwired: 2 in, 2 out]
    n121 = property on="Number of active Koheras lines" class="DigNum (strict)"() -> ("Value"=w376:i8)  [unwired: 2 in, 2 out]
    n122 = property on="Wavelength" class="Arr (strict)"() -> ("Value"=w379:i32[])  [unwired: 2 in, 2 out]
    n123 = case shown="\"Area\"" "Measurement Type" {
      tunnel: "Start" -> [_ _ w457]
      tunnel: w426 -> [_ _ w456]
      tunnel: w421 -> [_ _ w455]
      tunnel: w415 -> [_ _ w454]
      tunnel: w414 -> [_ _ w453]
      tunnel: w409 -> [_ _ w452]
      tunnel: w399 -> [_ _ w451]
      tunnel: w376 -> [_ _ w450]
      tunnel: w371 -> [_ _ w449]
      tunnel: w368 -> [_ _ w448]
      frame #0 {
      }
      frame #1 {
      }
      frame #2 {
        n124 = case shown="True" w457 {
          tunnel: w456 -> [_ w466]
          tunnel: w455 -> [_ w465]
          tunnel: w453 -> [_ w464]
          tunnel: w454 -> [_ w463]
          tunnel: w449 -> [_ w462]
          tunnel: w452 -> [_ w461]
          tunnel: w451 -> [_ w460]
          tunnel: w450 -> [_ w459]
          tunnel: w448 -> [_ w458]
          frame #0 {
          }
          frame #1 {
            n125 = stacked-sequence {
              tunnel: w466 -> [_ w509 w556 _]
              tunnel: w465 -> [_ w521 _ _]
              tunnel: w464 -> [_ w501 _ _]
              tunnel: w463 -> [_ w516 _ _]
              tunnel: w462 -> [_ w498 _ _]
              tunnel: w461 -> [_ w502 _ _]
              tunnel: w460 -> [_ w499 _ _]
              tunnel: w459 -> [_ w477 _ _]
              tunnel: w458 -> [_ w476 w523 _]
              frame #0 {
              }
              frame #1 {
                # "Running Measurement"
                n126 = Increment(x=w501) -> (x+1=w515:u8)
                n127 = Multiply(x=w516, y=w515) -> (x*y=w517:dbl)
                n128 = property on="Pulse per Wavelength" class="Arr (strict)"() -> ("Value"=w500:u8[])  [unwired: 2 in, 2 out]
                n129 = property on="Power settings" class="Arr (strict)"() -> ("Value"=w504:dbl[][])  [unwired: 2 in, 2 out]
                n130 = Unbundle(w476) -> ("AOTF-Digital switch in"=w475:tag, "Picture Clock out"=w474:tag, "AOTF-Analog switch in"=w473:tag, "Picture Clock Main out"=w472:tag, "Picture Start Clock in"=w471:tag, "Picture Clock Main in"=w470:tag, "Blanking Out"=w469:tag, "Delayed  Main Start Clock in"=w468:tag, "AOTF-Digital out"=w467:tag)
                n131 = call "AOTF_Digital_Pulse_Switch.vi"("Number of active lines"=w477, "AOTF-Digital out"=w467, "AOTF-Digital switch in"=w475, "Pictures per pixel"=w501, "Pulse per Wavelength"=w500) -> ("error out"=w513:errorcluster, "task out"=w510:refnum<k21>)  [unwired: 1 in, 4 out]
                n132 = call "AOTF_Analog_Pulse_Switch.vi"("Array 2"=w504, "Number of active lines"=w477, "AOTF-Analog out"=w509, "AOTF-Digital switch in"=w473, "Pictures per pixel"=w501, "Pulse per Wavelength"=w500) -> ("error out"=w508:errorcluster, "task out"=w505:refnum<k21>)  [unwired: 4 out]
                n133 = Unbundle(w499) -> ("Delay / [us]"=w492:i32, "Delayed Startclock out"=w491:tag, "Main Startclock In"=w490:tag, "20 MHz-Clock"=w489:tag)
                n134 = call "Pixel_Trigger_Main.vi"("Counter(s)"=w474, "Number Of Pulses"=w501, "Frequency"=w517, "Source"=w468) -> ("error out"=w514:errorcluster, "task out"=w518:refnum<k21>)  [unwired: 6 out]
                n135 = call "Timing_Main_Pulse_Delay.vi"("Source of Ticks"=w489, "Trigger Source"=w490, "Counter(s)"=w491, "Delay / [us]"=w492) -> ("error out"=w478:errorcluster, "task out"=w493:refnum<k21>)  [unwired: 6 out]
                n136 = call "Picture_Clock_Main.vi"("Picture-Time / [ms]"=w502, "Source"=w471, "Counter(s)"=w472) -> ("error out"=w479:errorcluster, "Number of Pulses per Picture / [x1 us]"=w485:i32, "task out"=w488:refnum<k21>)  [unwired: 1 in, 5 out]
                n137 = call <vilib>:"Merge Errors.vi"("error in 3 (no error)"=w508, "error in 2 (no error)"=w513, "error in 1 (no error)"=w514) -> ("error out"=w503:errorcluster)  [unwired: 1 in, 3 out]
                n138 = call <vilib>:"Merge Errors.vi"("error in 3 (no error)"=w478, "error in 2 (no error)"=w479, "error in 1 (no error)"=w503) -> ("error out"=w497:errorcluster)  [unwired: 1 in, 3 out]
                n139 = call <vilib>:"Merge Errors.vi"("error in 1 (no error)"=w497) -> ("error out"=w496:errorcluster)  [unwired: 3 in, 3 out]
                n140 = property on="Exposure Time" class="Arr (strict)"() -> ("Value"=w484:u32[][])  [unwired: 2 in, 2 out]
                n141 = call "Scanner_Ansteuerung_Main.vi"("error in"=w496, "Scanner Out-Ports"=w498, "Scanner Properties"=w521) -> ("error out"=w480:errorcluster)  [unwired: 7 in, 1 out]
                n142 = call "Picture_Exposure_Time.vi"("Pulse per Wavelength"=w500, "Exposure Time"=w484, "Blanking Out"=w469, "Picture Clock Main in"=w470, "Number of Pulses per Picture / [x1 us]"=w485, "Number of active Koheras lines"=w477) -> ("task out"=w481:refnum<k21>)  [unwired: 5 out]
                n143 = call <vilib>:"DAQmx Stop Task.vi"("task/channels in"=w518, "error in"=w480) -> ("task out"=w519:refnum<k21>, "error out"=w520:errorcluster)  [unwired: 12 out]
                n144 = call <vilib>:"DAQmx Stop Task.vi"("task/channels in"=w510, "error in"=w480) -> ("task out"=w512:refnum<k21>, "error out"=w511:errorcluster)  [unwired: 12 out]
                n145 = call <vilib>:"DAQmx Stop Task.vi"("task/channels in"=w505, "error in"=w480) -> ("task out"=w507:refnum<k21>, "error out"=w506:errorcluster)  [unwired: 12 out]
                n146 = call <vilib>:"DAQmx Stop Task.vi"("task/channels in"=w488, "error in"=w480) -> ("task out"=w487:refnum<k21>, "error out"=w486:errorcluster)  [unwired: 12 out]
                n147 = call <vilib>:"DAQmx Stop Task.vi"("task/channels in"=w493, "error in"=w480) -> ("task out"=w495:refnum<k21>, "error out"=w494:errorcluster)  [unwired: 12 out]
                n148 = call <vilib>:"DAQmx Stop Task.vi"("task/channels in"=w481, "error in"=w480) -> ("task out"=w483:refnum<k21>, "error out"=w482:errorcluster)  [unwired: 12 out]
                n149 = call <vilib>:"DAQmx Clear Task.vi"("task in"=w519, "error in"=w520) -> ()  [unwired: 14 out]
                n150 = call <vilib>:"DAQmx Clear Task.vi"("task in"=w512, "error in"=w511) -> ()  [unwired: 14 out]
                n151 = call <vilib>:"DAQmx Clear Task.vi"("task in"=w507, "error in"=w506) -> ()  [unwired: 14 out]
                n152 = call <vilib>:"DAQmx Clear Task.vi"("task in"=w487, "error in"=w486) -> ()  [unwired: 14 out]
                n153 = call <vilib>:"DAQmx Clear Task.vi"("task in"=w495, "error in"=w494) -> ()  [unwired: 14 out]
                n154 = call <vilib>:"DAQmx Clear Task.vi"("task in"=w483, "error in"=w482) -> ()  [unwired: 14 out]
              }
              frame #2 {
                w525 = 0 ("dimension size")
                w537 = 1 items=["one channel for each line", "one channel for all lines"] ("line grouping")
                w539 = 2 ("samples per channel")
                w538 = 1000.0 ("rate")
                w540 = 10178 items=["Finite Samples"=10178, "Continuous Samples"=10123, "Hardware Timed Single Point"=12522] ("sample mode")
                # "AOTF-Power-Configure - Switch AOTF-Power OFF"
                n155 = Unbundle(w523) -> ("AOTF-Digital out"=w522:tag)  [unwired: 8 out]
                n156 = call "AOTF_Create_analog_Ports.vi"("Cluster"=w556) -> ("task out"=w542:refnum<k21>, "error out"=w541:errorcluster)
                n157 = Initialize Array(0 ("dimension size"), 8 ("dimension size")) -> (w553:i32[])
                n158 = Build Array(w553, w553) -> (w543:i32[][])
                n159 = Transpose 2D Array(2D array=w543) -> (transposed array=w544:i32[][])
                n160 = call-poly <vilib>:"DAQmx Timing.vi"("task/channels in"=w542, "sample mode"=w540, "samples per channel"=w539, "rate"=w538, "error in"=w541) -> ("task out"=w552:refnum<k21>, "error out"=w551:errorcluster)  [unwired: 2 in, 7 out]
                n161 = call-poly <vilib>:"DAQmx Write.vi"("task/channels in"=w552, "data"=w544, "error in"=w551) -> ("task out"=w546:refnum<k21>, "error out"=w545:errorcluster)  [unwired: 1 in, 10 out]
                n162 = call-poly <vilib>:"DAQmx Create Virtual Channel.vi"("lines"=w522, "line grouping"=w537) -> ("task out"=w536:refnum<k21>, "error out"=w535:errorcluster)  [unwired: 3 in, 9 out]
                n163 = call <vilib>:"DAQmx Start Task.vi"("task/channels in"=w546, "error in"=w545) -> ("task out"=w547:refnum<k21>, "error out"=w548:errorcluster)  [unwired: 12 out]
                n164 = call-poly <vilib>:"DAQmx Timing.vi"("task/channels in"=w536, "sample mode"=w540, "samples per channel"=w539, "rate"=w538, "source"=tag "/Dev2/20MHzTimebase", "error in"=w535) -> ("task out"=w534:refnum<k21>, "error out"=w533:errorcluster)  [unwired: 1 in, 7 out]
                n165 = call <vilib>:"DAQmx Wait Until Done.vi"("task/channels in"=w547, "error in"=w548) -> ("task out"=w550:refnum<k21>, "error out"=w549:errorcluster)  [unwired: 1 in, 11 out]
                n166 = call <vilib>:"DAQmx Clear Task.vi"("task in"=w550, "error in"=w549) -> ()  [unwired: 14 out]
                n167 = Build Array(w525, w525) -> (w524:i32[])
                n168 = call-poly <vilib>:"DAQmx Write.vi"("task/channels in"=w534, "data"=w524, "error in"=w533) -> ("task out"=w528:refnum<k21>, "error out"=w527:errorcluster)  [unwired: 1 in, 10 out]
                n169 = call <vilib>:"DAQmx Start Task.vi"("task/channels in"=w528, "error in"=w527) -> ("task out"=w529:refnum<k21>, "error out"=w530:errorcluster)  [unwired: 12 out]
                n170 = call <vilib>:"DAQmx Wait Until Done.vi"("task/channels in"=w529, "error in"=w530) -> ("task out"=w532:refnum<k21>, "error out"=w531:errorcluster)  [unwired: 1 in, 11 out]
                n171 = call <vilib>:"DAQmx Clear Task.vi"("task in"=w532, "error in"=w531) -> ()  [unwired: 14 out]
              }
              frame #3 {
              }
            }
          }
        }
      }
    }
    n172 = case shown="\"Measurement\", Default" "?" {
      tunnel: "Koheras Seed Laser" -> [w581 _ w716 _ _ _ _]
      tunnel: w395 -> [w573 _ w709 _ _ _ _]
      tunnel: [w580 0 w708 0 0 0 0] -> w396
      tunnel: w394 -> [w576 _ w707 _ _ _ _]
      tunnel: w393 -> [w577 _ w706 _ _ _ _]
      tunnel: "Koheras-AOTF-Controller" -> [_ w637 w705 _ _ _ _]
      tunnel: w379 -> [_ w635 _ _ _ _ _]
      tunnel: [0 1 0 0 0 0 0] -> w378
      tunnel: w377 -> [_ w638 _ _ _ _ _]
      tunnel: w376 -> [_ w622 _ _ _ _ _]
      tunnel: w373 -> [_ w634 _ _ _ _ _]
      tunnel: [T5 {"Value"=0, "Value"=[], "Value"=[], "Set Manual"=FALSE} w633 T5 {"Value"=0, "Value"=[], "Value"=[], "Set Manual"=FALSE} T5 {"Value"=0, "Value"=[], "Value"=[], "Set Manual"=FALSE} T5 {"Value"=0, "Value"=[], "Value"=[], "Set Manual"=FALSE} T5 {"Value"=0, "Value"=[], "Value"=[], "Set Manual"=FALSE} T5 {"Value"=0, "Value"=[], "Value"=[], "Set Manual"=FALSE}] -> w375
      tunnel: w374 -> [_ w632 _ _ _ _ _]
      tunnel: w371 -> [_ _ _ w913 _ _ _]
      frame #0 {
        n173 = call "Koheras_Init.vi"("VISA resource name"=w581) -> ("VISA resource name out"=w579:refnum<visa-resource-name>, "error out"=w578:errorcluster)
        n174 = case shown="0, Default" w573 {
          tunnel: w579 -> [w589 w606]
          tunnel: w578 -> [w588 w605]
          tunnel: [w586 w604] -> _
          tunnel: [w587 w603] -> _
          tunnel: [0 1] -> w580
          tunnel: w576 -> [w584 _]
          tunnel: w577 -> [w583 _]
          tunnel: string[] ["get serialno", "get fwrev", "get disprev", "get hwrev", "get almb", "get alm", "get interlock", "get errorcode", "get dcs1", "get dcs2", "get dcs3", "get dc1", "get dc2", "get dc3", "get pd5", "get sensor0", "get sensor1", "get sensor2", "get sensor3", "get datetime", "get state", "get power", "get current"] -> [_ w594]
          tunnel: i32[] [18, 12, 14, 11, 26, 13, 13, 13, 10, 10, 10, 7, 7, 7, 7, 14, 14, 14, 14, 25, 9, 9, 11] -> [_ w592]
          frame #0 {
            n175 = call "Koheras_get_set_Status.vi"("error in"=w588, "Answer-Length"=w583, "Command in"=w584, "VISA resource name in"=w589) -> ("error out"=w587:errorcluster, "VISA resource name out"=w586:refnum<visa-resource-name>)  [unwired: 6 out]
          }
          frame #1 {
            n176 = Array Subset(array=w594, index=20, length=3) -> (w593:string[])
            n177 = Array Subset(array=w592, index=20, length=3) -> (w591:i32[])
            n178 = call "Koheras_get_set_Status.vi"("error in"=w605, "Answer-Length"=w591, "Command in"=w593, "VISA resource name in"=w606) -> ("error out"=w603:errorcluster, "Return"=w609:string[], "VISA resource name out"=w604:refnum<visa-resource-name>)  [unwired: 5 out]
            n179 = Index Array(array=w609, index #1=0 ("index"), index #2=1 ("index"), index #3=2 ("index")) -> (element #1=w600:string, element #2=w599:string, element #3=w598:string)
            n180 = Decimal String To Number(string=w598, offset=0) -> ()  [unwired: 3 out]
            n181 = Decimal String To Number(string=w600, offset=0) -> (number=w597:i32)  [unwired: 2 out]
            n182 = Decimal String To Number(string=w599, offset=0) -> (number=→"Actual Power Level / [%]":i32)  [unwired: 2 out]
            n183 = Not Equal?(x=w597, y=0) -> (x != y?=→"?":bool)
          }
        }
        n184 = property class="TabCtl (strict)"("Val(Sgnl)"="Laser Power Type") -> ()  [unwired: 2 in, 2 out]
      }
      frame #1 {
        n185 = case shown="1" w638 {
          tunnel: w637 -> [w701 w702]
          tunnel: [w701 w702] -> w636
          frame #0 {
            n186 = call "Koheras_AOTF-Init.vi"("Koheras-AOTF-Controller"=w701) -> ()  [unwired: 11 out]
          }
          frame #1 {
          }
        }
        n187 = Bundle("Value"=w622, "Value"=w635, "Value"=w634, "Set Manual"="Set Manual") -> (w633:T5)  [unwired: 1 out]
        n188 = Not Equal?(x=w633, y=w632) -> (x != y?=w630:T21)
        n189 = Unbundle(w630) -> ("Value"=w619:bool, "Value"=w627:bool[], "Value"=w620:bool[], "Set Manual"=w621:bool)
        n190 = property on="Number of active Koheras lines" class="DigNum (strict)"("Val(Sgnl)"="Number of active Koheras lines") -> ()  [unwired: 2 in, 2 out]
        n191 = Boolean Array To Number(Boolean array=w620) -> (number=w629:u32)
        n192 = Boolean Array To Number(Boolean array=w627) -> (number=w628:u32)
        n193 = Add(x=w629, y=w628) -> (x+y=w626:u32)
        n194 = Not Equal?(x=w626, y=u32 0) -> (x != y?=w624:bool)
        n195 = Or(x=w621, y=w624) -> (x .or. y?=w618:bool)
        n196 = Or(x=w618, y=w619) -> (x .or. y?=w617:bool)
        n197 = case shown="True" w617 {
          tunnel: w636 -> [_ w647]
          tunnel: w635 -> [_ w646]
          tunnel: w634 -> [_ w645]
          tunnel: "Set Manual" -> [_ w644]
          tunnel: w622 -> [_ w642]
          frame #0 {
            n198 = property on="Programming AOTF" class="Bool (strict)"("Val(Sgnl)"=FALSE ("Value (Signaling)")) -> ()  [unwired: 2 in, 2 out]
          }
          frame #1 {
            n199 = case shown="True" w644 {
              tunnel: w646 -> [_ w648]
              tunnel: w647 -> [_ w655]
              tunnel: w645 -> [_ w650]
              tunnel: w642 -> [_ w651]
              frame #0 {
              }
              frame #1 {
                w653 = 8
                n200 = Subtract(x=w653, y=w651) -> (x-y=w652:i32)
                n201 = for {
                  N: w653 -> [_]
                  tunnel: w655 -> [w686]
                  tunnel: [w686] -> w654
                  tunnel: w648 -> [w688] mode=indexing
                  i -> [w687]
                  w695 = FALSE ("replace all? (F)")
                  n202 = Number To Decimal String(number=w688) -> (decimal integer string=w690:string)  [unwired: 1 out]
                  n203 = Number To Decimal String(number=w687) -> (decimal integer string=w692:string)  [unwired: 1 out]
                  n204 = Concatenate Strings("dds frequency " ("string"), w692, " #" ("string"), w690, "\r") -> (w684:string)
                  n205 = call "Koheras_AOTF.vi"("String"=w684, "VISA resource name 2"=w686) -> ("read buffer"=w685:string)  [unwired: 9 out]
                  n206 = Search and Replace String(replace all?=w695, input string=w685, search string="\r\n", replace string="" ("replace string (\"\")")) -> (result string=w697:string)  [unwired: 1 in, 6 out]
                  n207 = Search and Replace String(replace all?=w695, input string=w697, search string="*" ("replace string (\"\")"), replace string="" ("replace string (\"\")")) -> (result string=→"Command":string)  [unwired: 1 in, 6 out]
                }
                n208 = for {
                  N: w652 -> [_]
                  tunnel: w651 -> [w661]
                  shift-right: [w659] -> w649
                  shift-left: w650 -> [w658]
                  i -> [w660]
                  n209 = Add(x=w661, y=w660) -> (x+y=w657:i32)
                  n210 = Replace Array Subset(array=w658, new element=0 ("new element/subarray"), index=w657) -> (w659:i32[])
                }
                n211 = for {
                  N: w653 -> [_]
                  tunnel: w654 -> [w664]
                  tunnel: w649 -> [w665] mode=indexing
                  i -> [w682]
                  w676 = FALSE ("replace all? (F)")
                  n212 = Divide(x=w665, y=100) -> (x/y=w673:dbl)
                  n213 = Multiply(x=16383, y=w673) -> (x*y=w671:dbl)
                  n214 = To Long Integer(number=w671) -> (32bit integer=w667:i32)
                  n215 = Number To Decimal String(number=w667) -> (decimal integer string=w669:string)  [unwired: 1 out]
                  n216 = Number To Decimal String(number=w682) -> (decimal integer string=w681:string)  [unwired: 1 out]
                  n217 = Concatenate Strings("dds amplitude " ("string"), w681, " " ("string"), w669, "\r") -> (w663:string)
                  n218 = call "Koheras_AOTF.vi"("String"=w663, "VISA resource name 2"=w664) -> ("read buffer"=w662:string)  [unwired: 9 out]
                  n219 = Search and Replace String(replace all?=w676, input string=w662, search string="\r\n", replace string="" ("replace string (\"\")")) -> (result string=w677:string)  [unwired: 1 in, 6 out]
                  n220 = Search and Replace String(replace all?=w676, input string=w677, search string="*" ("replace string (\"\")"), replace string="" ("replace string (\"\")")) -> (result string=w666:string)  [unwired: 1 in, 6 out]
                  n221 = property on="Command" class="Str"("Val(Sgnl)"=w666) -> ()  [unwired: 2 in, 2 out]
                }
              }
            }
            "Programming AOTF" <- TRUE ("Programming AOTF")
          }
        }
      }
      frame #2 {
        n222 = call "Koheras_Init.vi"("VISA resource name"=w716) -> ("VISA resource name out"=w715:refnum<visa-resource-name>, "error out"=w712:errorcluster)
        n223 = case shown="0, Default" w709 {
          tunnel: w715 -> [w762 w858 w865 w882]
          tunnel: string[] ["get serialno", "get fwrev", "get disprev", "get hwrev", "get almb", "get alm", "get interlock", "get errorcode", "get dcs1", "get dcs2", "get dcs3", "get dc1", "get dc2", "get dc3", "get pd5", "get sensor0", "get sensor1", "get sensor2", "get sensor3", "get datetime", "get state", "get power", "get current"] -> [w749 w823 _ w879]
          tunnel: i32[] [18, 12, 14, 11, 26, 13, 13, 13, 10, 10, 10, 7, 7, 7, 7, 14, 14, 14, 14, 25, 9, 9, 11] -> [w743 w825 _ w880]
          tunnel: w712 -> [w761 w857 w864 w881]
          tunnel: [w760 w856 w862 w878] -> w711
          tunnel: [w759 w855 w863 w877] -> w710
          tunnel: [1 3 1 1] -> w708
          tunnel: w707 -> [_ _ w860 _]
          tunnel: w706 -> [_ _ w859 _]
          tunnel: w705 -> [w722 _ _ _]
          frame #0 {
            n224 = Array Subset(array=w749, index=0, length=4) -> (w746:string[])
            n225 = Array Subset(array=w743, index=0, length=4) -> (w742:i32[])
            n226 = call "Koheras_get_set_Status.vi"("error in"=w761, "Answer-Length"=w742, "Command in"=w746, "VISA resource name in"=w762) -> ("error out"=w759:errorcluster, "Return"=w758:string[], "VISA resource name out"=w760:refnum<visa-resource-name>)  [unwired: 5 out]
            n227 = Build Array("BoardID ID" ("string"), "BoardID S" ("string"), "BoardID V" ("string")) -> (w718:string[])
            n228 = for {
              tunnel: [w770] -> w723
              tunnel: w722 -> [w769]
              shift-right: [w768] -> w724
              shift-left: "" -> [w766]
              tunnel: w718 -> [w765] mode=indexing
              n229 = Concatenate Strings(w765, "\r") -> (w763:string)
              n230 = call "Koheras_AOTF.vi"("String"=w763, "VISA resource name 2"=w769) -> ("error out"=w770:errorcluster, "read buffer"=w767:string)  [unwired: 8 out]
              n231 = Concatenate Strings(w766, w767) -> (w768:string)
            }
            n232 = Index Array(array=w758, index #1=0 ("index"), index #2=1 ("index"), index #3=2 ("index"), index #4=3 ("index")) -> (element #1=→"SuperK Serial No.":string, element #2=→"SuperK Firmware rev. Main":string, element #3=→"SuperK Firmware rev. Display":string, element #4=→"SuperK Firmware rev. Hardware":string)
            n233 = call <vilib>:"Clear Errors.vi"("error in (no error)"=w723) -> ("error out"=w735:errorcluster)  [unwired: 6 out]
            n234 = Search and Replace String(replace all?=TRUE ("replace all? (F)"), case sensitive?=FALSE ("ignore case? (F)"), input string=w724, search string="*", replace string=".*." ("replace string (\"\")"), offset=0 ("offset (0)"), error in=w735) -> (number of replacements=w734:i32)  [unwired: 4 out]
            n235 = for {
              N: w734 -> [_]
              shift-right: [w786] -> _
              shift-left: w724 -> [w784]
              tunnel: [w773] -> w727 mode=indexing
              w790 = "*" ("search string")
              n236 = Search and Replace String(replace all?=FALSE ("replace all? (F)"), case sensitive?=FALSE ("ignore case? (F)"), input string=w784, search string=w790, replace string=w790) -> (result string=w787:string, offset past replacement=w783:i32)  [unwired: 1 in, 4 out]
              n237 = Build Array("\r\n", "*" ("element"), "BoardID ID" ("string"), "BoardID S" ("string"), "BoardID V" ("string"), "Board ID:" ("string"), "Serial Number:" ("string")) -> (w779:string[])
              n238 = String Subset(string=w787, offset (0)=w783) -> (substring=w786:string)  [unwired: 1 out]
              n239 = Array Size(array=w779) -> (size(s)=w778:i32)
              n240 = String Subset(string=w784, offset (0)=0, length (rest)=w783) -> (substring=w781:string)
              n241 = for {
                N: w778 -> [_]
                tunnel: w779 -> [w792] mode=indexing
                shift-right: [w795] -> w774
                shift-left: w781 -> [w791]
                n242 = Search and Replace String(replace all?=TRUE ("replace all? (F)"), input string=w791, search string=w792, replace string="" ("replace string (\"\")")) -> (result string=w795:string)  [unwired: 1 in, 6 out]
              }
              n243 = call <vilib>:"Trim Whitespace.vi"("string"=w774) -> ("trimmed string"=w773:string)  [unwired: 1 in]
            }
            n244 = Rotate 1D Array(1:w727, 2:3 ("n")) -> (0:w726:string[])
            n245 = Index Array(array=w726, index=1) -> (element=→"Board Serial":string)
            n246 = Index Array(array=w726, index=2) -> (element=→"Board Version":string)
            n247 = Index Array(array=w726, index=0) -> (element=→"Board ID":string)
          }
          frame #1 {
            w837 = " °C" ("string")
            n248 = Array Subset(array=w823, index=11, length=8) -> (w827:string[])
            n249 = Array Subset(array=w825, index=11, length=8) -> (w835:i32[])
            n250 = Array Size(array=w827) -> (size(s)=w831:i32)
            n251 = Array Size(array=w835) -> (size(s)=w836:i32)
            n252 = Array Subset(array=w823, index=6, length=1) -> (w828:string[])
            n253 = Array Subset(array=w825, index=6, length=1) -> (w832:i32[])
            n254 = Insert Into Array(array=w827, index=w831, new element=w828) -> (w826:string[])
            n255 = Insert Into Array(array=w835, index=w836, new element=w832) -> (w824:i32[])
            n256 = call "Koheras_get_set_Status.vi"("error in"=w857, "Answer-Length"=w824, "Command in"=w826, "VISA resource name in"=w858) -> ("error out"=w855:errorcluster, "Return"=w813:string[], "VISA resource name out"=w856:refnum<visa-resource-name>)  [unwired: 5 out]
            n257 = Index Array(array=w813, index #1=4 ("index"), index #2=5 ("index"), index #3=6 ("index"), index #4=7 ("index"), index #5=8 ("index"), index #6=0 ("index"), index #7=1 ("index"), index #8=2 ("index"), index #9=3 ("index")) -> (element #1=w844:string, element #2=w842:string, element #3=w840:string, element #4=w838:string, element #5=w821:string, element #6=w804:string, element #7=w803:string, element #8=w802:string, element #9=w801:string)
            n258 = Concatenate Strings(w844, w837) -> (→"Temperature Seed Laser":string)
            n259 = Concatenate Strings(w842, w837) -> (→"Temperature Preamplifier":string)
            n260 = Concatenate Strings(w840, w837) -> (→"Temperature Booster":string)
            n261 = Concatenate Strings(w838, w837) -> (→"Temperature Case":string)
            n262 = Decimal String To Number(string=w804, offset=0) -> (number=w800:i32)  [unwired: 2 out]
            n263 = Decimal String To Number(string=w803, offset=0) -> (number=w799:i32)  [unwired: 2 out]
            n264 = Decimal String To Number(string=w802, offset=0) -> (number=w798:i32)  [unwired: 2 out]
            n265 = Decimal String To Number(string=w801, offset=0) -> (number=→"Output Photodiode current":i32)  [unwired: 2 out]
            n266 = Decimal String To Number(string=w821, offset=0) -> (number=w816:i32)  [unwired: 2 out]
            n267 = Bundle(w800, w799, w798) -> (→"Diode current":cluster{i32, i32, i32})  [unwired: 1 out]
            n268 = Equal?(x=w816, y=0) -> (x = y?=w818:bool)
            n269 = Equal?(x=w816, y=2) -> (x = y?=→"Reset Interlock":bool)
            n270 = Not(x=w818) -> (.not. x?=→"Interlock":bool)
          }
          frame #2 {
            n271 = call "Koheras_get_set_Status.vi"("error in"=w864, "Answer-Length"=w859, "Command in"=w860, "VISA resource name in"=w865) -> ("error out"=w863:errorcluster, "VISA resource name out"=w862:refnum<visa-resource-name>)  [unwired: 6 out]
          }
          frame #3 {
            n272 = Array Subset(array=w879, index=20, length=3) -> (w876:string[])
            n273 = Array Subset(array=w880, index=20, length=3) -> (w875:i32[])
            n274 = call "Koheras_get_set_Status.vi"("error in"=w881, "Answer-Length"=w875, "Command in"=w876, "VISA resource name in"=w882) -> ("error out"=w877:errorcluster, "Return"=w885:string[], "VISA resource name out"=w878:refnum<visa-resource-name>)  [unwired: 5 out]
            n275 = Index Array(array=w885, index #1=0 ("index"), index #2=1 ("index"), index #3=2 ("index")) -> (element #1=w872:string, element #2=w871:string, element #3=w870:string)
            n276 = Decimal String To Number(string=w870, offset=0) -> ()  [unwired: 3 out]
            n277 = Decimal String To Number(string=w872, offset=0) -> (number=w869:i32)  [unwired: 2 out]
            n278 = Decimal String To Number(string=w871, offset=0) -> (number=→"Actual Power Level / [%]":i32)  [unwired: 2 out]
            n279 = Not Equal?(x=w869, y=0) -> (x != y?=→"?":bool)
          }
        }
        n280 = VISA Close(VISA resource name=w711, error in (no error)=w710) -> ()  [unwired: 1 out]
      }
      frame #3 {
        w922 = 10178 items=["Finite Samples"=10178, "Continuous Samples"=10123, "Hardware Timed Single Point"=12522] ("sample mode")
        n281 = Unbundle(w913) -> ("Analog-Channel X"=w912:tag, "Analog-Channel Y"=w911:tag)  [unwired: 2 out]
        n282 = case shown="False" "Set Manual" {
          tunnel: "X-Voltage" -> [_ w929]
          tunnel: "Y-Voltage" -> [_ w928]
          tunnel: [0.0 ("X-Voltage") w929] -> w895
          tunnel: [0.0 ("Y-Voltage") w928] -> w894
          frame #0 {
          }
          frame #1 {
          }
        }
        n283 = call-poly <vilib>:"DAQmx Create Virtual Channel.vi"("maximum value"=10.0, "minimum value"=0.0, "physical channels"=w912) -> ("task out"=w916:refnum<k21>, "error out"=w917:errorcluster)  [unwired: 6 in, 5 out]
        n284 = call-poly <vilib>:"DAQmx Create Virtual Channel.vi"("task in"=w916, "maximum value"=10.0, "minimum value"=0.0, "physical channels"=w911, "error in"=w917) -> ("task out"=w914:refnum<k21>, "error out"=w915:errorcluster)  [unwired: 4 in, 5 out]
        n285 = Build Array(w895, w895) -> (w899:dbl[])
        n286 = Build Array(w894, w894) -> (w896:dbl[])
        n287 = Build Array(w899, w896) -> (w898:dbl[][])
        n288 = call-poly <vilib>:"DAQmx Timing.vi"("task/channels in"=w914, "sample mode"=w922, "samples per channel"=2, "rate"=1000.0, "error in"=w915) -> ("task out"=w901:refnum<k21>, "error out"=w900:errorcluster)  [unwired: 2 in, 7 out]
        n289 = call-poly <vilib>:"DAQmx Write.vi"("task/channels in"=w901, "data"=w898, "error in"=w900) -> ("task out"=w903:refnum<k21>, "error out"=w902:errorcluster)  [unwired: 2 in, 9 out]
        n290 = call <vilib>:"DAQmx Start Task.vi"("task/channels in"=w903, "error in"=w902) -> ("task out"=w904:refnum<k21>, "error out"=w905:errorcluster)  [unwired: 12 out]
        n291 = call <vilib>:"DAQmx Wait Until Done.vi"("task/channels in"=w904, "error in"=w905) -> ("task out"=w907:refnum<k21>, "error out"=w906:errorcluster)  [unwired: 1 in, 11 out]
        n292 = call <vilib>:"DAQmx Clear Task.vi"("task in"=w907, "error in"=w906) -> ()  [unwired: 14 out]
      }
      frame #4 {
      }
      frame #5 {
      }
      frame #6 {
      }
    }
    n293 = property on="stop" class="Bool (strict)"() -> ("Value"=w437:bool)  [unwired: 2 in, 2 out]
    "Running" <- "Start"
    "active 9" <- "PicoQuant Laser Head"
    "?" <- "PicoQuant Laser Head"
  }
  n294 = call-poly <vilib>:"DAQmx Create Virtual Channel.vi"("frequency"=1.0 ("Frequency 2"), "duty cycle"=0.1 ("Duty Cycle"), "counter"="Clock out", "idle state"=w18, "initial delay"=0.0) -> ("task out"=w22:refnum<k21>, "error out"=w23:errorcluster)  [unwired: 4 in, 5 out]
  n295 = flat-sequence {
    tunnel: [w940] -> w4
    tunnel: w3 -> [w939]
    frame #0 {
      w947 = u16 5 items=["9600", "14400", "19200", "38400", "57600", "115200"] ("Baudrate")
      w942 = u16 0 items=["RS232", "GPIB"] ("Interface")
      n296 = Bundle("PI E710"="PI E710", "Baudrate"=w947) -> (w948:cluster{"PI E710":u16, "Baudrate":u16})  [unwired: 1 out]
      n297 = call <userlib>:"E710_Configuration_Setup.vi"("System no."=w939, "Are stages connected?"=bool[] [TRUE, TRUE, TRUE, FALSE, FALSE, FALSE], "Change servo \nstatus to ON?"=TRUE ("Change servo \nstatus to ON?"), "Perform autozero?"=FALSE ("All axes?"), "Interface"=w942, "RS232 settings"=w948, "Move to middle?"=FALSE) -> ("error out"=w940:errorcluster)  [unwired: 5 in, 7 out]
    }
  }
  n298 = while {
    tunnel: w3 -> [w950]
    shift-right: [w949] -> _
    shift-left: _ -> [w952]
    stop <- w951 stop-if-true
    n299 = case shown="False" "SCANNER EMERGENCY" {
      tunnel: w950 -> [_ w966]
      tunnel: w952 -> [w955 w968]
      tunnel: [w955 w967] -> w949
      frame #0 {
        n300 = Wait Until Next ms Multiple(millisecond multiple=u32 100) -> ()  [unwired: 1 out]
      }
      frame #1 {
        n301 = Build Array("wgo 10" ("String to send"), "wgo 20" ("String to send"), "wgo 30" ("String to send"), "wgo 10 20" ("String to send"), "wgo 10 30" ("String to send"), "wgo 20 30" ("String to send"), "wgo 10 20 30" ("String to send")) -> (w957:string[])
        n302 = for {
          N: 7 -> [_]
          tunnel: w968 -> [_]
          tunnel: w966 -> [w971]
          tunnel: [w970] -> w958
          tunnel: w957 -> [w969] mode=indexing
          n303 = call "PI_E710_Communicate.vi"("System no."=w971, "String to send"=w969) -> ("error out"=w970:errorcluster)  [unwired: 1 in, 8 out]
        }
        n304 = flat-sequence {
          tunnel: [w972] -> w967
          tunnel: w958 -> [w972]
          frame #0 {
            n305 = One Button Dialog(message="Emergency scanner stop appeared!!!\nCheck scanner settings before continue!!!") -> ()  [unwired: 2 out]
          }
        }
      }
    }
    n306 = property on="stop" class="Bool (strict)"() -> ("Value"=w951:bool)  [unwired: 2 in, 2 out]
  }
  n307 = while {
    shift-right: [w976] -> _
    shift-left: FALSE -> [w977]
    tunnel: w3 -> [w975]
    stop <- w976 stop-if-true
    # "Program-End Control Task"
    n308 = Wait Until Next ms Multiple(millisecond multiple=u32 100) -> ()  [unwired: 1 out]
    n309 = case shown="True" "stop" {
      selector: "stop" -> [_ w986]
      tunnel: [w981 w986] -> w976
      tunnel: w977 -> [w981 _]
      tunnel: w975 -> [_ w984]
      tunnel: [errorcluster {"status"=FALSE, "code"=0, "source"=""} ("error out") w983] -> _
      tunnel: [errorcluster {"status"=FALSE, "code"=0, "source"=""} ("error out") w982] -> _
      frame #0 {
      }
      frame #1 {
        n310 = call <userlib>:"Close connection if open.vi"("System no."=w984) -> ("error out"=w983:errorcluster)  [unwired: 1 in, 17 out]
        n311 = Wait Until Next ms Multiple(millisecond multiple=u32 100) -> ()  [unwired: 1 out]
        n312 = call "ShutDown.vi"() -> ("error out"=w982:errorcluster)  [unwired: 1 in, 2 out]
      }
    }
  }
  n313 = call-poly <vilib>:"DAQmx Timing.vi"("task/channels in"=w22, "sample mode"=w19, "error in"=w23) -> ("task out"=w20:refnum<k21>, "error out"=w21:errorcluster)  [unwired: 3 in, 8 out]
  n314 = call-poly <vilib>:"DAQmx Create Virtual Channel.vi"("lines"="Power Driver", "line grouping"=w28) -> ("task out"=w32:refnum<k21>, "error out"=w31:errorcluster)  [unwired: 3 in, 9 out]
  n315 = call "Heidenhain_Init.vi"("VISA resource name"="Heidenhain_Seriell") -> ("VISA resource name out"=w38:refnum<visa-resource-name>, "error out"=w37:errorcluster)
  n316 = call <vilib>:"DAQmx Start Task.vi"("task/channels in"=w20, "error in"=w21) -> ("task out"=w13:refnum<k21>, "error out"=w12:errorcluster)  [unwired: 12 out]
  n317 = call <vilib>:"DAQmx Start Task.vi"("task/channels in"=w32, "error in"=w31) -> ("task out"=w30:refnum<k21>, "error out"=w29:errorcluster)  [unwired: 12 out]
  n318 = while {
    tunnel: w38 -> [w1050]
    tunnel: w37 -> [w1049]
    tunnel: [w1048] -> w44
    tunnel: [w1047] -> w43
    shift-right: [w989] -> _
    shift-left: 0.0 ("default value 1") -> [w1046]
    tunnel: w30 -> [w1043]
    tunnel: w29 -> [w1042]
    tunnel: [w1040] -> w25
    tunnel: [w1039] -> w24
    tunnel: w13 -> [w1035]
    tunnel: w12 -> [w1033]
    tunnel: [w1032] -> w11
    tunnel: [w1034] -> w10
    shift-right: [w1027] -> _
    shift-left: w8 -> [w1031]
    shift-left: w8 -> [w1026]
    shift-right: [w995] -> _
    shift-left: 0 -> [w1024]
    shift-right: [w1022] -> _
    shift-left: 0 -> [w1023]
    shift-right: [w988] -> _
    shift-left: _ -> [w1016]
    shift-right: ["Fix Position"] -> _
    shift-left: _ -> [w1015]
    shift-right: ["Choose Position"] -> _
    shift-left: _ -> [w994]
    stop <- w1044 stop-if-true
    n319 = Equal?(x=w1031, y=w1026) -> (x = y?=w1030:bool[])
    n320 = property on="Running" class="Bool (strict)"() -> ("Value"=w1051:bool)  [unwired: 2 in, 2 out]
    n321 = Wait Until Next ms Multiple(millisecond multiple=u32 1000) -> ()  [unwired: 1 out]
    n322 = Boolean Array To Number(Boolean array=w1030) -> (number=w1029:u32)
    n323 = case shown="False" w1051 {
      tunnel: w1050 -> [w1089 w1092]
      tunnel: w1049 -> [w1088 w1091]
      tunnel: [w1087 w1092] -> w1048
      tunnel: [w1086 w1091] -> w1047
      tunnel: [w1085 w1090] -> w989
      tunnel: w1046 -> [_ w1090]
      frame #0 {
        # "z-Position- Control"
        # "Haidenhain-Probe Control"
        n324 = call "Heidenhain_Read.vi"("VISA resource name out"=w1089, "error out"=w1088) -> ("VISA resource name out 2"=w1087:refnum<visa-resource-name>, "default value 1"=w1085:dbl, "error IO"=w1086:errorcluster)
      }
      frame #1 {
        # "Interupted during Measurement"
      }
    }
    "Actual Microscope Position / [mm]" <- w989
    n325 = Equal?(x=w1029, y=u32 15) -> (x = y?=w1025:bool)
    n326 = case shown="True" w1025 {
      tunnel: w1024 -> [_ w1082]
      tunnel: [0 ("y") w1078] -> w1017
      frame #0 {
      }
      frame #1 {
        w1077 = 4000 ("y")
        n327 = Add(x=w1082, y=100) -> (x+y=w1079:i32)
        n328 = Greater Or Equal?(x=w1079, y=w1077) -> (x >= y?=w1080:bool)
        n329 = case shown="False" w1080 {
          tunnel: w1079 -> [w1083 _]
          tunnel: [w1083 w1084] -> w1078
          tunnel: w1077 -> [_ w1084]
          frame #0 {
          }
          frame #1 {
          }
        }
      }
    }
    n330 = Less?(x=w1015, y="Fix Position") -> (x < y?=w1013:bool)
    n331 = Or(x=w1013, y="Reset Fix Position") -> (x .or. y?=w993:bool)
    n332 = case shown="False" w993 {
      tunnel: w989 -> [_ w1063]
      tunnel: [w1062 w1063] -> w992
      tunnel: w1016 -> [w1062 _]
      frame #0 {
      }
      frame #1 {
      }
    }
    n333 = Not Equal?(x=w994, y="Choose Position") -> (x != y?=w991:bool)
    n334 = case shown="False" w991 {
      tunnel: w992 -> [w1052 _]
      tunnel: [w1052 w1053] -> w988
      tunnel: "Choose Position" -> [_ w1053]
      frame #0 {
      }
      frame #1 {
      }
    }
    "Fixed Position / [mm]" <- w988
    n335 = Greater?(x=w989, y=w988) -> (0:w1012:bool)
    n336 = Less?(x=w989, y=w988) -> (x < y?=w1011:bool)
    n337 = Subtract(x=w989, y=w988) -> (x-y=w1003:dbl)
    n338 = Subtract(x=w989, y=w988) -> (x-y=→"Differenz":dbl)
    n339 = And(x=w1012, y="Fix Position") -> (x .and. y?=w1007:bool)
    n340 = And(x=w1011, y="Fix Position") -> (x .and. y?=w1008:bool)
    n341 = Absolute Value(x=w1003) -> (abs(x)=w1000:dbl)
    n342 = Or(x=w1007, y="Move Down") -> (x .or. y?=w1006:bool)
    n343 = Or(x=w1008, y="Move Up") -> (x .or. y?=w1009:bool)
    n344 = Multiply(x=100000.0, y=w1000) -> (x*y=w996:dbl)
    n345 = Or(x=w1009, y=w1006) -> (x .or. y?=w1020:bool)
    n346 = Less Or Equal?(x=w996, y=4000.0) -> (x <= y?=w997:bool)
    n347 = case shown="True" w1020 {
      tunnel: [0 ("y") w1075] -> w1004
      tunnel: w1017 -> [_ w1075]
      frame #0 {
      }
      frame #1 {
      }
    }
    n348 = case shown="False" w1020 {
      tunnel: w1023 -> [w1069 _]
      tunnel: [w1066 0] -> w1022
      tunnel: [w1064 FALSE] -> w1021
      frame #0 {
        w1067 = 10 ("y")
        n349 = Add(x=w1069, y=1) -> (x+y=w1065:i32)
        n350 = Greater Or Equal?(x=w1065, y=w1067) -> (x >= y?=w1064:bool)
        n351 = case shown="False" w1064 {
          tunnel: w1067 -> [_ w1071]
          tunnel: [w1070 w1071] -> w1066
          tunnel: w1065 -> [w1070 _]
          frame #0 {
          }
          frame #1 {
          }
        }
      }
      frame #1 {
      }
    }
    n352 = And(x=w997, y="Fix Position") -> (x .and. y?=w998:bool)
    n353 = case shown="False" w998 {
      tunnel: w1004 -> [w1054 _]
      tunnel: [w1054 w1058] -> w995
      tunnel: w996 -> [_ w1057]
      frame #0 {
      }
      frame #1 {
        n354 = Greater?(x=w1057, y="Numeric 2") -> (0:w1056:bool)
        n355 = case shown="False" w1056 {
          tunnel: w1057 -> [_ w1061]
          tunnel: [w1059 w1060] -> w1058
          tunnel: "Numeric 2" -> [w1059 _]
          frame #0 {
          }
          frame #1 {
            n356 = To Long Integer(number=w1061) -> (32bit integer=w1060:i32)
          }
        }
      }
    }
    "Numeric" <- w995
    n357 = Build Array("Clutch", w1006, w1021, w1020) -> (w1027:bool[])
    n358 = Boolean Array To Number(Boolean array=w1027) -> (number=w1037:u32)
    n359 = Divide(x=w995, y=40) -> (x/y=→"Moving Speed / [%]":dbl)
    n360 = Build Array(w1037) -> (w1036:u32[])
    n361 = property class="DAQmx Channel"(reference=w1035, error in=w1033, "CO.Pulse.Freq"=w995) -> (reference out=w1034:refnum<k21>, error out=w1032:errorcluster)
    n362 = call-poly <vilib>:"DAQmx Write.vi"("task/channels in"=w1043, "auto start"=TRUE, "data"=w1036, "error in"=w1042) -> ("task out"=w1040:refnum<k21>, "error out"=w1039:errorcluster)  [unwired: 10 out]
    n363 = property on="stop" class="Bool (strict)"() -> ("Value"=w1044:bool)  [unwired: 2 in, 2 out]
  }
  n364 = while {
    tunnel: w4 -> [w1112]
    tunnel: w3 -> [w1111]
    shift-right: [w1105] -> _
    shift-left: w2 -> [w1104]
    shift-left: w2 -> [w1103]
    shift-right: [w1097] -> _
    shift-left: T4 {"", "cancelled"=FALSE, "error out"={"status"=FALSE, "code"=0, "source"=""}, FALSE, "Slides"=0, ""} -> [w1098]
    stop <- w1117 stop-if-true
    n365 = flat-sequence {
      tunnel: [w1171] -> w1108
      frame #0 {
        n366 = property on="Intensity Graph" class="IntGraph (strict)"() -> ("Cursor.Cursor X"=w1166:dbl)  [unwired: 2 in, 2 out]
        n367 = property on="Intensity Graph" class="IntGraph (strict)"() -> ("Cursor.Cursor Y"=w1164:dbl)  [unwired: 2 in, 2 out]
        n368 = Less Or Equal To 0?(x=w1166) -> (x <= 0?=w1165:bool)
        n369 = Less Or Equal To 0?(x=w1164) -> (x <= 0?=w1163:bool)
        n370 = case shown="True" w1165 {
          tunnel: w1166 -> [w1174 _]
          tunnel: [w1174 1] -> w1170
          frame #0 {
          }
          frame #1 {
          }
        }
        n371 = case shown="True" w1163 {
          tunnel: w1164 -> [w1172 _]
          tunnel: [w1172 1] -> w1168
          frame #0 {
          }
          frame #1 {
          }
        }
        n372 = To Word Integer(number=w1170) -> (16bit integer=→"Cursor X":i16)
        n373 = To Word Integer(number=w1168) -> (16bit integer=→"Cursor Y":i16)
        n374 = Bundle("Cursor.Cursor X"=w1170, "Cursor.Cursor Y"=w1168) -> (w1171:T22)  [unwired: 1 out]
      }
    }
    n375 = flat-sequence {
      tunnel: w1104 -> [w1144]
      tunnel: w1103 -> [w1147]
      tunnel: [w1143] -> w1102
      frame #0 {
        n376 = Unbundle(w1144) -> ("Boolean array"=w1148:bool[])  [unwired: 10 out]
        n377 = Unbundle(w1147) -> ("Boolean array"=w1146:bool[])  [unwired: 10 out]
        n378 = Index Array(array=w1148, index=7) -> (element=w1150:bool)
        n379 = Index Array(array=w1146, index=7) -> (element=w1152:bool)
        n380 = Not Equal?(x=w1150, y=w1152) -> (x != y?=w1149:bool)
        n381 = case shown="True" w1149 {
          tunnel: w1148 -> [w1157 w1159]
          tunnel: [w1154 w1158] -> w1145
          frame #0 {
            n382 = Replace Array Subset(array=w1157, new element=FALSE ("new element/subarray"), index=6) -> (w1154:bool[])
          }
          frame #1 {
            w1162 = 10 ("element")
            n383 = Replace Array Subset(array=w1159, new element=TRUE ("new element/subarray"), index=6) -> (w1158:bool[])
            n384 = property on="Intensity Graph" class="IntGraph (strict)"("Cursor.Cursor X"=w1162) -> ()  [unwired: 2 in, 2 out]
            n385 = property on="Intensity Graph" class="IntGraph (strict)"("Cursor.Cursor Y"=w1162) -> ()  [unwired: 2 in, 2 out]
          }
        }
        n386 = Bundle(cluster=w1144, "Boolean array"=w1145) -> (w1143:T14)  [unwired: 10 out]
      }
    }
    n387 = case shown="\"Picture\", Default" "Measurement Mode" {
      tunnel: [TRUE ("Visible") w1224 TRUE ("Visible")] -> w1114
      tunnel: w1108 -> [_ w1217 w1327]
      tunnel: [TRUE ("ROI") TRUE ("ROI") "ROI"] -> w1113
      tunnel: w1112 -> [_ w1215 w1323]
      tunnel: w1111 -> [_ w1214 w1322]
      tunnel: w1102 -> [w1198 w1207 w1318]
      tunnel: [w1198 w1205 w1309] -> w1107
      tunnel: [w1197 w1204 w1311] -> w1096
      tunnel: "Exposure time / ms" -> [_ w1203 w1307]
      tunnel: w1098 -> [w1196 w1202 w1295]
      tunnel: [w1196 w1202 w1294] -> w1097
      frame #0 {
        n388 = Wait (ms)(milliseconds to wait=100) -> ()  [unwired: 1 out]
        n389 = Unbundle(w1198) -> (w1197:i32[][])  [unwired: 10 out]
      }
      frame #1 {
        n390 = flat-sequence {
          tunnel: [w1228] -> _
          tunnel: ["upper right 2"] -> _
          tunnel: ["lower left 2"] -> _
          tunnel: [w1229] -> _
          tunnel: [w1225] -> w1211
          frame #0 {
            w1240 = 128 ("dimension size")
            w1241 = 1 ("dimension size")
            n391 = Bundle("dimension size"=w1241, "dimension size"=w1241, "dimension size"=w1240, "dimension size"=w1240) -> (w1228:T12)  [unwired: 1 out]
            n392 = Bundle("x- lower left"="x- lower left", "y- lower left"="y- lower left", "x- upper right"="x- upper right", "y-upper right"="y-upper right") -> (w1229:T23)  [unwired: 1 out]
            n393 = Unbundle(w1229) -> ("x- lower left"=w1231:u8, "y- lower left"=w1234:u8, "x- upper right"=w1230:u8, "y-upper right"=w1236:u8)
            n394 = Bundle(w1229, w1228, "lower left 2"="lower left 2", "upper right 2"="upper right 2") -> (w1225:T24)  [unwired: 1 out]
            n395 = Subtract(x=w1230, y=w1231) -> (x-y=→"X-Pixels":u8)
            n396 = Subtract(x=w1236, y=w1234) -> (x-y=→"Y-Pixels":u8)
          }
        }
        n397 = case shown="\"Int Trace\"" "?" {
          tunnel: [TRUE ("Visible") FALSE ("Visible") TRUE ("Visible")] -> w1224
          frame #0 {
          }
          frame #1 {
          }
          frame #2 {
          }
        }
        n398 = Build Array("x-Position", "y-Position", "z-Position") -> (w1220:dbl[])
        n399 = case shown="\"Stage\", Default" "?" {
          tunnel: w1220 -> [_ w1277]
          tunnel: w1215 -> [w1275 w1287]
          tunnel: w1214 -> [_ w1288]
          tunnel: w1207 -> [w1274 w1280]
          tunnel: [w1275 w1282] -> _
          tunnel: [w1274 w1279] -> w1206
          frame #0 {
          }
          frame #1 {
            n400 = Unbundle(w1280) -> (w1278:cluster{dbl[], dbl[]})  [unwired: 10 out]
            n401 = Bundle(cluster=w1278, w1277) -> (w1276:cluster{dbl[], dbl[]})  [unwired: 1 out]
            n402 = Unbundle(w1278) -> (w1281:dbl[])  [unwired: 1 out]
            n403 = Not Equal?(x=w1281, y=w1277) -> (x != y?=w1290:bool[])
            n404 = Bundle(cluster=w1280, w1276) -> (w1279:T14)  [unwired: 10 out]
            n405 = property on="actual scan stage position" class="Arr (strict)"() -> ("Value"=w1285:dbl[])  [unwired: 2 in, 2 out]
            n406 = Boolean Array To Number(Boolean array=w1290) -> (number=w1289:u32)
            n407 = Equal To 0?(x=w1289) -> (x = 0?=w1286:bool)
            n408 = property class="Bool (strict)"() -> ("Value"=w1284:bool)  [unwired: 2 in, 2 out]
            n409 = call "Position_show_and_move.vi"("Target position"=w1277, "Measurement running"=w1284, "error in"=w1287, "System no."=w1288, "Move"=w1286, "actual scan position"=w1285) -> ("error out"=w1282:errorcluster, "Value"=→"actual scan stage position":dbl[])  [unwired: 4 out]
          }
        }
        n410 = case shown="False" "Zoom" {
          tunnel: w1217 -> [w1263 _]
          tunnel: [w1261 w1272] -> w1212
          tunnel: w1211 -> [w1262 w1273]
          frame #0 {
            n411 = Unbundle(w1262) -> (w1261:T12, "lower left 2"=w1260:bool, "upper right 2"=w1259:bool)  [unwired: 1 out]
            n412 = case shown="True" w1260 {
              tunnel: w1263 -> [_ w1267]
              frame #0 {
              }
              frame #1 {
                n413 = Unbundle(w1267) -> ("Cursor.Cursor X"=w1266:dbl, "Cursor.Cursor Y"=w1265:dbl)
                n414 = property on="x- lower left" class="DigNum (strict)"("Val(Sgnl)"=w1266) -> (error out=w1264:errorcluster)  [unwired: 2 in, 1 out]
                n415 = property on="y- lower left" class="DigNum (strict)"(error in=w1264, "Val(Sgnl)"=w1265) -> ()  [unwired: 1 in, 2 out]
              }
            }
            n416 = case shown="True" w1259 {
              tunnel: w1263 -> [_ w1271]
              frame #0 {
              }
              frame #1 {
                n417 = Unbundle(w1271) -> ("Cursor.Cursor X"=w1268:dbl, "Cursor.Cursor Y"=w1270:dbl)
                n418 = property on="y-upper right" class="DigNum (strict)"("Val(Sgnl)"=w1270) -> (error out=w1269:errorcluster)  [unwired: 2 in, 1 out]
                n419 = property on="x- upper right" class="DigNum (strict)"(error in=w1269, "Val(Sgnl)"=w1268) -> ()  [unwired: 1 in, 2 out]
              }
            }
          }
          frame #1 {
            n420 = Unbundle(w1273) -> (w1272:T23)  [unwired: 3 out]
          }
        }
        n421 = flat-sequence {
          tunnel: [w1247] -> w1209
          tunnel: w1206 -> [w1244]
          tunnel: w1203 -> [w1242]
          frame #0 {
            n422 = call "Picture_Accquire.vi"("Input Cluster 2"=w1244, "Accquire"="Accquire") -> ("output cluster"=w1243:T14, "New Value"=→"?":bool)  [unwired: 1 in, 7 out]
            n423 = call "Andor_iXon_Init_Update_Exposuretime.vi"("Input Cluster"=w1243, "Num of Pictures"="Num of Pictures", "Exposure time / ms"=w1242) -> ("output cluster"=w1247:T14)  [unwired: 8 out]
          }
        }
        n424 = call "Andor_iXon_Point-mode.vi"("Input Cluster 2"=w1209, "Enum"="?", "Cluster"=w1212) -> ("Output Cluster"=w1205:T14, "Numeric"=w1208:dbl)  [unwired: 7 out]
        n425 = flat-sequence {
          tunnel: w1208 -> [w1256]
          tunnel: w1205 -> [w1250]
          tunnel: "?" -> [w1255]
          frame #0 {
            n426 = Unbundle(w1250) -> ("Boolean array"=w1249:bool[])  [unwired: 10 out]
            n427 = Index Array(array=w1249, index=7) -> (element=w1253:bool)
            n428 = Equal?(x=w1255, y=enum32{"Picture", "Int Trace", "Video"}."Int Trace") -> (x = y?=w1252:bool)
            n429 = And(x=w1252, y=w1253) -> (x .and. y?=w1251:bool)
            n430 = case shown="True" w1251 {
              tunnel: w1256 -> [_ w1258]
              frame #0 {
              }
              frame #1 {
                "Waveform Chart 2" <- w1258
              }
            }
          }
        }
        n431 = Unbundle(w1205) -> (w1204:i32[][])  [unwired: 10 out]
        n432 = call "Picture_Save_to_matlab.vi"("Input Cluster"=w1205, "Mode"="?", "Save"="Save") -> ()  [unwired: 9 out]
      }
      frame #2 {
        n433 = flat-sequence {
          tunnel: [w1445] -> w1308
          frame #0 {
            n434 = Bundle("left limit"="left limit", "lower limit"="lower limit", "x-Pixel"="x-Pixel", "y-Pixel"="y-Pixel") -> (w1444:T25)  [unwired: 1 out]
            n435 = case shown="True" "Square" {
              tunnel: w1444 -> [_ w1451]
              frame #0 {
              }
              frame #1 {
                n436 = Unbundle(w1451) -> ("x-Pixel"=w1450:i32)  [unwired: 3 out]
                n437 = property on="y-Pixel" class="DigNum (strict)"("Val(Sgnl)"=w1450) -> ()  [unwired: 2 in, 2 out]
              }
            }
            n438 = call "Picture_Square_ROI.vi"("Square"="Square", "Cluster"=w1444) -> ("Cluster 2"=w1445:T26)  [unwired: 9 out]
            "?" <- "Square"
          }
        }
        n439 = Unbundle(w1327) -> ("Cursor.Cursor X"=w1325:dbl, "Cursor.Cursor Y"=w1326:dbl)
        n440 = flat-sequence {
          tunnel: w1318 -> [w1466]
          tunnel: [w1464] -> w1300
          frame #0 {
            n441 = Bundle("x-Pixel"="x-Pixel", "y-Pixel"="y-Pixel", "x-Position"="x-Position", "y-Position"="y-Position", "Picture size"="Picture size", "?", "?", "z-Position"="z-Position") -> (w1467:T6)  [unwired: 1 out]
            n442 = Unbundle(w1467) -> ("Picture size"=→"?":dbl, →"?":dbl)  [unwired: 6 out]
            n443 = call "Picture_Square_Pixel.vi"("input cluster"=w1467, "Square"="Square") -> ("Output Cluster"=w1465:T6)  [unwired: 1 in, 8 out]
            n444 = Bundle(cluster=w1466, "cluster"=w1465) -> (w1464:T14)  [unwired: 10 out]
            n445 = case shown="True" "Square" {
              tunnel: w1465 -> [_ w1481]
              frame #0 {
              }
              frame #1 {
                n446 = Unbundle(w1481) -> ("y-Pixel"=w1480:u16, w1479:dbl)  [unwired: 6 out]
                n447 = property on="y-Pixel" class="DigNum (strict)"("Val(Sgnl)"=w1480) -> ()  [unwired: 2 in, 2 out]
                n448 = property class="DigNum (strict)"("Val(Sgnl)"=w1479) -> ()  [unwired: 2 in, 2 out]
              }
            }
            "?" <- "Square"
          }
        }
        n449 = Wait (ms)(milliseconds to wait=100) -> ()  [unwired: 1 out]
        n450 = case shown="True" "Accquire" {
          tunnel: [w1336 w1341] -> w1302
          tunnel: "Stack?" -> [w1335 w1338]
          tunnel: w1295 -> [w1336 w1339]
          tunnel: [w1333 w1338] -> w1298
          tunnel: "Accquire" -> [w1332 w1337]
          tunnel: [w1332 w1337] -> w1296
          frame #0 {
            n451 = property class="Boolesch (strikt)"() -> ("Value"=w1334:bool)  [unwired: 2 in, 2 out]
            n452 = And(x=w1335, y=w1334) -> (x .and. y?=w1333:bool)
          }
          frame #1 {
            n453 = case shown="True" w1338 {
              selector: w1338 -> [_ w1349]
              tunnel: [w1343 w1350] -> w1341
              tunnel: "Slides" -> [_ w1348]
              tunnel: w1339 -> [w1343 _]
              frame #0 {
              }
              frame #1 {
                n454 = File Dialog(4:"MatLab" ("pattern label"), 6:"*.mat" ("pattern (all files)")) -> (0:w1345:errorcluster, 1:w1346:bool, 3:w1347:path)  [unwired: 1 in, 5 out]
                n455 = Path To String(path=w1347) -> (string=w1344:string)
                n456 = Bundle(w1344, "cancelled"=w1346, "error out"=w1345, w1349, "Slides"=w1348, w1344) -> (w1350:T4)  [unwired: 1 out]
              }
            }
            n457 = property on="Slide" class="DigitalWert (strikt)"("Value"=0 ("Slide")) -> ()  [unwired: 2 in, 2 out]
            "?" <- w1338
          }
        }
        n458 = case shown="True" "lower left" {
          tunnel: w1325 -> [_ w1714]
          tunnel: w1326 -> [_ w1713]
          frame #0 {
          }
          frame #1 {
            n459 = property on="left limit" class="DigNum (strict)"("Val(Sgnl)"=w1714) -> ()  [unwired: 2 in, 2 out]
            n460 = property on="lower limit" class="DigNum (strict)"("Val(Sgnl)"=w1713) -> ()  [unwired: 2 in, 2 out]
          }
        }
        n461 = case shown="True" "upper right" {
          tunnel: w1326 -> [_ w1709]
          tunnel: w1325 -> [_ w1712]
          frame #0 {
          }
          frame #1 {
            n462 = property on="left limit" class="DigNum (strict)"() -> ("Value"=w1711:i32)  [unwired: 2 in, 2 out]
            n463 = property on="lower limit" class="DigNum (strict)"() -> ("Value"=w1708:i32)  [unwired: 2 in, 2 out]
            n464 = Subtract(x=w1712, y=w1711) -> (x-y=w1710:dbl)
            n465 = Subtract(x=w1709, y=w1708) -> (x-y=w1707:dbl)
            n466 = property on="x-Pixel" class="DigNum (strict)"("Val(Sgnl)"=w1710) -> ()  [unwired: 2 in, 2 out]
            n467 = property on="y-Pixel" class="DigNum (strict)"("Val(Sgnl)"=w1707) -> ()  [unwired: 2 in, 2 out]
          }
        }
        n468 = case shown="True" w1298 {
          tunnel: w1296 -> [w1355 _]
          tunnel: [w1355 w1384] -> w1303
          tunnel: [w1354 w1382] -> w1294
          tunnel: w1302 -> [w1354 w1370]
          tunnel: w1300 -> [w1353 w1381]
          tunnel: [w1353 w1380] -> w1299
          frame #0 {
          }
          frame #1 {
            n469 = Unbundle(w1381) -> ("cluster"=w1379:T6)  [unwired: 10 out]
            n470 = property on="Slide" class="DigitalWert (strikt)"() -> ("Value"=w1361:i32)  [unwired: 2 in, 2 out]
            n471 = Unbundle(w1370) -> (w1368:string, "Slides"=w1362:i32)  [unwired: 4 out]
            n472 = Wait (ms)(milliseconds to wait=u32 2000 ("Zu wartende ms")) -> ()  [unwired: 1 out]
            n473 = Greater Or Equal?(x=w1361, y=w1362) -> (x >= y?=w1383:bool)
            n474 = Less?(x=w1361, y=w1362) -> (x < y?=w1384:bool)
            n475 = Increment(x=w1361) -> (x+1=w1363:i32)
            "Slide" <- w1363
            n476 = String Length(string=w1368) -> (length=w1367:i32)
            n477 = Unbundle(w1379) -> ("x-Position"=w1376:dbl, "y-Position"=w1375:dbl, w1377:enum32{"x-y", "x-z", "y-z"}, "z-Position"=w1374:dbl)  [unwired: 4 out]
            n478 = case shown="True" w1383 {
              frame #0 {
              }
              frame #1 {
                n479 = property class="Boolesch (strikt)"("Val(Sgnl)"=FALSE ("Wert (signalisierend)")) -> ()  [unwired: 2 in, 2 out]
              }
            }
            n480 = Subtract(x=w1367, y=5) -> (x-y=w1365:i32)
            n481 = Divide(x="Step-width [nm]", y=1000) -> (x/y=w1371:dbl)
            n482 = Number To Decimal String(number=w1363) -> (decimal integer string=w1359:string)  [unwired: 1 out]
            n483 = case shown="\"y-z\"" w1377 {
              tunnel: w1379 -> [w1389 w1394 w1398]
              tunnel: [w1388 w1393 w1399] -> w1378
              tunnel: w1376 -> [_ _ w1397]
              tunnel: w1375 -> [_ w1392 _]
              tunnel: w1374 -> [w1387 _ _]
              tunnel: w1371 -> [w1386 w1391 w1396]
              frame #0 {
                n484 = Add(x=w1387, y=w1386) -> (x+y=w1385:dbl)
                n485 = property on="z-Position" class="DigitalWert (strikt)"("Val(Sgnl)"=w1385) -> ()  [unwired: 2 in, 2 out]
                n486 = Bundle(cluster=w1389, "z-Position"=w1385) -> (w1388:T6)  [unwired: 7 out]
              }
              frame #1 {
                n487 = Add(x=w1392, y=w1391) -> (x+y=w1390:dbl)
                n488 = property on="y-Position" class="DigitalWert (strikt)"("Val(Sgnl)"=w1390) -> ()  [unwired: 2 in, 2 out]
                n489 = Bundle(cluster=w1394, "y-Position"=w1390) -> (w1393:T6)  [unwired: 7 out]
              }
              frame #2 {
                n490 = Add(x=w1397, y=w1396) -> (x+y=w1395:dbl)
                n491 = property on="x-Position" class="DigitalWert (strikt)"("Val(Sgnl)"=w1395) -> ()  [unwired: 2 in, 2 out]
                n492 = Bundle(cluster=w1398, "x-Position"=w1395) -> (w1399:T6)  [unwired: 7 out]
              }
            }
            n493 = Search/Split String(string=w1368, search string/char (-)="." ("Nach String/Zeichen suchen (-)"), offset (0)=w1365) -> (substring before match=w1364:string, match + rest of string=w1360:string)  [unwired: 1 out]
            n494 = Concatenate Strings(w1364, "-" ("Nach String/Zeichen suchen (-)"), w1359, w1360) -> (w1356:string)
            n495 = Bundle(cluster=w1370, w1356) -> (w1382:T4)  [unwired: 5 out]
            n496 = Bundle(cluster=w1381, "cluster"=w1378) -> (w1380:T14)  [unwired: 10 out]
          }
        }
        n497 = call "PI_Scanrange_limit.vi"("Input Cluster"=w1299, "Enum"="?") -> ("Output Cluster"=w1317:T14)  [unwired: 2 in, 7 out]
        n498 = flat-sequence {
          tunnel: w1317 -> [w1453]
          frame #0 {
            n499 = Unbundle(w1453) -> ("cluster"=w1452:T6)  [unwired: 10 out]
            n500 = Unbundle(w1452) -> ("x-Pixel"=w1460:u16, "y-Pixel"=w1461:u16, "Picture size"=w1455:dbl, w1454:dbl)  [unwired: 4 out]
            n501 = property class="DigNum (strict)"("Val(Sgnl)"=w1454) -> ()  [unwired: 2 in, 2 out]
            n502 = Divide(x=w1455, y=w1460) -> (x/y=w1463:dbl)
            n503 = Divide(x=w1454, y=w1461) -> (x/y=w1462:dbl)
            n504 = property on="Picture size" class="DigNum (strict)"("Val(Sgnl)"=w1455) -> ()  [unwired: 2 in, 2 out]
            n505 = Multiply(x=w1463, y=1000.0) -> (x*y=→"x":dbl)
            n506 = Multiply(x=w1462, y=1000.0) -> (x*y=→"y":dbl)
          }
        }
        n507 = call "Picture_Init_Size.vi"("Input Cluster"=w1317) -> ("Output Cluster"=w1319:T14, "Boolean"=w1320:bool)  [unwired: 9 out]
        n508 = case shown="True" w1320 {
          frame #0 {
          }
          frame #1 {
            w1442 = 10.0 ("Cursor.Cursor Position:Cursor X")
            n509 = property on="Intensity Graph" class="IntGraph (strict)"("Cursor.Cursor X"=w1442) -> ()  [unwired: 2 in, 2 out]
            n510 = property on="Intensity Graph" class="IntGraph (strict)"("Cursor.Cursor Y"=w1442) -> ()  [unwired: 2 in, 2 out]
          }
        }
        n511 = case shown="\"Stage\", Default" "?" {
          tunnel: w1323 -> [w1501 _]
          tunnel: w1322 -> [w1499 _]
          tunnel: w1303 -> [w1491 _]
          tunnel: w1319 -> [w1489 w1706]
          tunnel: [w1487 w1706] -> w1315
          tunnel: w1307 -> [w1486 _]
          frame #0 {
            n512 = call "PI_Picture_dyn_scanner_prepare.vi"("Input Cluster"=w1489) -> ("Measurement time / [s]"=w1485:u32, "Commandset out"=w1504:string[])  [unwired: 9 out]
            n513 = Unbundle(w1489) -> ("Boolean array"=w1493:bool[], w1503:cluster{dbl[], dbl[]})  [unwired: 9 out]
            n514 = Unbundle(w1503) -> (w1502:dbl[])  [unwired: 1 out]
            n515 = Index Array(array=w1493, index=7) -> (element=w1495:bool)
            n516 = call "Picture_switch_value.vi"("Boolean array in"=w1493, "Value to switch"=7, "Switch"=w1491) -> ("Boolean array out"=w1494:bool[], "New Value"=→"?":bool)  [unwired: 7 out]
            n517 = property on="actual scan stage position" class="Arr (strict)"() -> ("Value"=w1498:dbl[])  [unwired: 2 in, 2 out]
            n518 = call "Position_show_and_move.vi"("Target position"=w1502, "Measurement running"=w1495, "error in"=w1501, "System no."=w1499, "Move"=FALSE, "actual scan position"=w1498) -> ("error out"=w1500:errorcluster, "Value"=w1497:dbl[])  [unwired: 4 out]
            n519 = Multiply(x=w1485, y="Scanner Divider") -> (x*y=w1484:u32)
            "Measurement time / [s]" <- w1484
            n520 = Bundle(cluster=w1489, "Boolean array"=w1494) -> (w1488:T14)  [unwired: 10 out]
            n521 = case shown="True" w1491 {
              tunnel: w1500 -> [_ w1539]
              tunnel: w1499 -> [_ w1538]
              tunnel: w1504 -> [_ w1516]
              tunnel: w1488 -> [w1505 w1529]
              tunnel: [w1505 w1531] -> w1487
              tunnel: w1486 -> [_ w1527]
              tunnel: w1484 -> [_ w1537]
              tunnel: "Scanner Divider" -> [_ w1506]
              frame #0 {
              }
              frame #1 {
                w1522 = 0 ("Index (Zeile)")
                # "Start Measurement"
                n522 = call "Andor_iXon_Init_Picture_Prepare.vi"("Output Cluster"=w1529, "Exposure time / ms"=w1527) -> ("output cluster"=w1528:T14)
                n523 = Number To Decimal String(number=w1506) -> (decimal integer string=w1507:string)  [unwired: 1 in]
                n524 = Concatenate Strings("SPA 1 0X13000109 " ("Neues Element/Teil-Array"), w1507) -> (w1508:string)
                n525 = Insert Into Array(array=w1516, index=2, new element="ccl 1 advanced" ("Neues Element/Teil-Array")) -> (w1518:string[])
                n526 = Insert Into Array(array=w1518, index=3, new element=w1508) -> (w1515:string[])
                n527 = stacked-sequence {
                  tunnel: w1539 -> [w1554 w1621 _ _ _ _ _]
                  tunnel: w1538 -> [w1555 w1622 _ _ w1640 _ _]
                  tunnel: w1515 -> [w1550 w1619 _ _ _ _ _]
                  tunnel: [_ _ _ _ w1644 _ _] -> _
                  tunnel: w1528 -> [w1553 _ w1633 _ w1643 w1660 _]
                  tunnel: w1527 -> [_ _ _ _ _ _ _]
                  tunnel: [_ _ w1635 _ _ _ _] -> _
                  tunnel: [_ _ w1636 _ _ _ _] -> _
                  tunnel: [_ _ _ _ _ w1662 _] -> _
                  tunnel: [_ _ _ _ _ w1661 _] -> w1533
                  tunnel: w1537 -> [w1552 _ _ _ _ w1659 _]
                  frame #0 {
                    n528 = case shown="True" "Learning loop" {
                      tunnel: w1555 -> [_ w1586]
                      tunnel: w1554 -> [_ w1585]
                      tunnel: w1550 -> [_ w1583]
                      tunnel: w1553 -> [_ w1571]
                      tunnel: w1552 -> [_ w1562]
                      frame #0 {
                      }
                      frame #1 {
                        w1563 = u16 35 ("Value")
                        w1574 = "0X13000003 " ("string")
                        # "Preparing Scanner"
                        n529 = Unbundle(w1571) -> ("cluster"=w1573:T6)  [unwired: 10 out]
                        n530 = Array Subset(array=w1583, index=2 ("Index"), length=6 ("Länge")) -> (w1580:string[])
                        n531 = Unbundle(w1573) -> ("y-Pixel"=w1565:u16, w1572:enum32{"x-y", "x-z", "y-z"})  [unwired: 6 out]
                        n532 = case shown="\"x-y\", Default" w1572 {
                          tunnel: ["WGO 1193 2449" ("String to send") "WGO 1193 3449" ("String to send") "WGO 2193 3449" ("String to send")] -> w1570
                          frame #0 {
                          }
                          frame #1 {
                          }
                          frame #2 {
                          }
                        }
                        n533 = Divide(x=w1562, y=w1565) -> (x/y=w1564:dbl)
                        n534 = Number To Decimal String(number=1 ("Wert")) -> (decimal integer string=w1577:string)  [unwired: 1 out]
                        n535 = property on="Programming scanner" class="Slide (strict)"("Caption.Text"="Preparing Scanner" ("Beschriftung.Text")) -> (error out=w1559:errorcluster)  [unwired: 2 in, 1 out]
                        n536 = call "PI_SPA.vi"("Value"=w1563, "Register"=w1574, "Axis"=w1577, "Commandset in"=w1580) -> ("Commandset out"=w1578:string[])  [unwired: 7 out]
                        n537 = Multiply(x=w1564, y=w1563) -> (x*y=w1561:dbl)
                        n538 = Number To Decimal String(number=2 ("Wert")) -> (decimal integer string=w1575:string)  [unwired: 1 out]
                        n539 = call "PI_SPA.vi"("Value"=w1563, "Register"=w1574, "Axis"=w1575, "Commandset in"=w1578) -> ("Commandset out"=w1569:string[])  [unwired: 7 out]
                        n540 = Array Size(array=w1569) -> (size(s)=w1568:i32)
                        n541 = for {
                          N: w1568 -> [w1610]
                          tunnel: w1586 -> [w1613]
                          tunnel: w1585 -> [w1616]
                          tunnel: [w1615] -> w1584
                          tunnel: w1569 -> [w1614] mode=indexing
                          tunnel: [w1613] -> w1567
                          tunnel: w1559 -> [_]
                          i -> [w1612]
                          n542 = call "PI_E710_Communicate.vi"("error out 2"=w1616, "System no."=w1613, "String to send"=w1614) -> ("error out"=w1615:errorcluster)  [unwired: 8 out]
                          n543 = Increment(x=w1612) -> (x+1=w1611:i32)
                          n544 = Divide(x=w1611, y=w1610) -> (x/y=w1609:dbl)
                          n545 = Multiply(x=100.0, y=w1609) -> (x*y=w1607:dbl)
                          n546 = property on="Programming scanner" class="Slide (strict)"("Value"=w1607) -> ()  [unwired: 2 in, 2 out]
                        }
                        n547 = call "PI_E710_Communicate.vi"("error out 2"=w1584, "System no."=w1567, "String to send"=w1570) -> ("error out"=w1558:errorcluster)  [unwired: 8 out]
                        n548 = property on="Programming scanner" class="Slide (strict)"(error in=w1558, "Caption.Text"="Learning Loop" ("Beschriftung.Text")) -> (error out=w1556:errorcluster)  [unwired: 1 in, 1 out]
                        n549 = Tick Count (ms)() -> (millisecond timer value=w1566:u32)
                        n550 = while {
                          tunnel: w1556 -> [w1593]
                          tunnel: w1567 -> [w1592]
                          tunnel: w1561 -> [w1595]
                          tunnel: w1566 -> [w1596]
                          tunnel: [w1591] -> _
                          stop <- w1587 stop-if-true
                          n551 = Tick Count (ms)() -> (millisecond timer value=w1602:u32)
                          n552 = call <userlib>:"#9.vi"("System no."=w1592, "error in"=w1593) -> ("WG running?"=w1590:bool[], "error out"=w1591:errorcluster)  [unwired: 16 in]
                          n553 = Wait (ms)(milliseconds to wait=u32 500 ("Zu wartende ms")) -> ()  [unwired: 1 out]
                          n554 = Subtract(x=w1602, y=w1596) -> (x-y=w1601:u32)
                          n555 = Boolean Array To Number(Boolean array=w1590) -> (number=w1589:u32)
                          n556 = Equal?(x=w1589, y=u32 0) -> (x = y?=w1587:bool)
                          n557 = Divide(x=w1601, y=u32 1000) -> (x/y=w1597:dbl)
                          n558 = Divide(x=w1597, y=w1595) -> (x/y=w1599:dbl)
                          n559 = Multiply(x=w1599, y=100.0) -> (x*y=w1594:dbl)
                          n560 = property on="Programming scanner" class="Slide (strict)"("Val(Sgnl)"=w1594) -> ()  [unwired: 2 in, 2 out]
                        }
                      }
                    }
                  }
                  frame #1 {
                    # "Preparing Scanner"
                    n561 = Array Size(array=w1619) -> (size(s)=w1620:i32)
                    n562 = property on="Programming scanner" class="Schieberegler (strikt)"("Caption.Text"="Preparing Scanner" ("Beschriftung.Text")) -> (error out=w1617:errorcluster)  [unwired: 2 in, 1 out]
                    n563 = for {
                      N: w1620 -> [w1626]
                      tunnel: w1622 -> [w1629]
                      tunnel: w1621 -> [w1632]
                      tunnel: [w1631] -> _
                      tunnel: w1619 -> [w1630] mode=indexing
                      tunnel: [w1629] -> _
                      tunnel: w1617 -> [_]
                      i -> [w1628]
                      n564 = call "PI_E710_Communicate.vi"("error out 2"=w1632, "System no."=w1629, "String to send"=w1630) -> ("error out"=w1631:errorcluster)  [unwired: 8 out]
                      n565 = Increment(x=w1628) -> (x+1=w1627:i32)
                      n566 = Divide(x=w1627, y=w1626) -> (x/y=w1625:dbl)
                      n567 = Multiply(x=100.0, y=w1625) -> (x*y=→"Programming scanner":dbl)
                    }
                  }
                  frame #2 {
                    n568 = call "Andor_iXon_Init_Picture.vi"("Input Cluster 2"=w1633) -> ("Output Cluster"=w1635:T14)  [unwired: 10 out]
                    n569 = Unbundle(w1635) -> (w1634:T13)  [unwired: 10 out]
                    n570 = call "Andor_iXon_Init.vi"("input cluster"=w1634) -> ("error out"=w1637:errorcluster)  [unwired: 1 in, 9 out]
                    n571 = call "StartAcquisition.vi"("error in (no error)"=w1637) -> ("error out"=w1636:errorcluster)  [unwired: 2 out]
                  }
                  frame #3 {
                    n572 = Wait Until Next ms Multiple(millisecond multiple=u32 2000 ("Vielfache von ms")) -> ()  [unwired: 1 out]
                  }
                  frame #4 {
                    n573 = Unbundle(w1643) -> ("cluster"=w1642:T6)  [unwired: 10 out]
                    n574 = Unbundle(w1642) -> (w1641:enum32{"x-y", "x-z", "y-z"})  [unwired: 7 out]
                    n575 = case shown="\"x-y\", Default" w1641 {
                      tunnel: w1640 -> [_ _ _]
                      tunnel: ["WGO 1129 2385" ("String to send") "WGO 1129 3385" ("String to send") "WGO 2129 3385" ("String to send")] -> w1639
                      frame #0 {
                      }
                      frame #1 {
                      }
                      frame #2 {
                      }
                    }
                    n576 = call "PI_E710_Communicate.vi"("System no."=w1640, "String to send"=w1639) -> ("error out"=w1644:errorcluster)  [unwired: 1 in, 8 out]
                  }
                  frame #5 {
                    n577 = Unbundle(w1660) -> (w1654:T13, "cluster"=w1658:T6)  [unwired: 9 out]
                    n578 = Unbundle(w1658) -> ("x-Pixel"=w1653:u16, "y-Pixel"=w1652:u16)  [unwired: 6 out]
                    n579 = Initialize Array(0.0 ("index"), w1653, w1652) -> (w1655:dbl[][])
                    n580 = property on="Programming scanner" class="Schieberegler (strikt)"("Caption.Text"="Accquire Picture" ("Beschriftung.Text")) -> (error out=w1648:errorcluster)  [unwired: 2 in, 1 out]
                    n581 = Tick Count (ms)() -> (millisecond timer value=w1663:u32)
                    n582 = while {
                      tunnel: [w1700] -> w1664
                      tunnel: w1663 -> [w1697]
                      tunnel: w1659 -> [w1690]
                      tunnel: w1648 -> [_]
                      stop <- w1702 continue-if-true
                      w1703 = u16 72  # DRV ACQUIRING
                      n583 = Tick Count (ms)() -> (millisecond timer value=w1698:u32)
                      n584 = Wait (ms)(milliseconds to wait=u32 500 ("Zu wartende ms")) -> ()  [unwired: 1 out]
                      n585 = Subtract(x=w1698, y=w1697) -> (x-y=w1696:u32)
                      n586 = call "GetStatus.vi"() -> ("error out"=w1700:errorcluster, "status"=w1701:T27)  [unwired: 1 in, 3 out]
                      n587 = Divide(x=w1696, y=u32 1000) -> (x/y=w1691:dbl)
                      n588 = Equal?(x=w1701, y=w1703) -> (x = y?=w1702:bool)
                      n589 = Divide(x=w1691, y=w1690) -> (x/y=w1694:dbl)
                      n590 = Multiply(x=w1694, y=100.0) -> (x*y=w1692:dbl)
                      n591 = property on="Programming scanner" class="Schieberegler (strikt)"("Val(Sgnl)"=w1692) -> ()  [unwired: 2 in, 2 out]
                    }
                    n592 = call "Andor_iXon_GetData.vi"("error in"=w1664, "input cluster"=w1654) -> ("error out"=w1662:errorcluster, "Array 3"=w1666:i32[][][], "array"=w1651:i32[])  [unwired: 2 in, 5 out]
                    n593 = Array Size(array=w1666) -> (size(s)=w1668:i32[])
                    n594 = Index Array(array=w1668, index=0) -> (element=w1665:i32)
                    n595 = for {
                      N: w1665 -> [_]
                      tunnel: w1666 -> [w1677] mode=indexing
                      tunnel: [w1678] -> w1650 mode=indexing
                      n596 = case shown="True" "Average or max.\nIntensity" {
                        tunnel: [w1679 w1688] -> w1678
                        tunnel: w1677 -> [w1680 w1681]
                        frame #0 {
                          n597 = Array Max & Min(array=w1680) -> (max value=w1679:i32)  [unwired: 3 out]
                        }
                        frame #1 {
                          n598 = Add Array Elements(numeric array=w1681) -> (sum=w1689:i32)
                          n599 = Array Size(array=w1681) -> (size(s)=w1685:i32[])
                          n600 = Index Array(array=w1685, index=0 ("Index")) -> (element=w1683:i32)
                          n601 = Index Array(array=w1685, index=1 ("Index")) -> (element=w1682:i32)
                          n602 = Multiply(x=w1683, y=w1682) -> (x*y=w1684:i32)
                          n603 = Divide(x=w1689, y=w1684) -> (x/y=w1688:dbl)
                        }
                      }
                    }
                    n604 = for {
                      N: w1652 -> [_]
                      tunnel: w1653 -> [w1672]
                      shift-right: [w1674] -> w1656
                      shift-left: w1655 -> [w1675]
                      tunnel: w1650 -> [w1670]
                      i -> [w1669]
                      n605 = Multiply(x=w1672, y=w1669) -> (x*y=w1673:i32)
                      n606 = Array Subset(array=w1670, index=w1673, length=w1672) -> (w1671:dbl[])
                      n607 = Replace Array Subset(array=w1675, new element=w1671, index (col)=w1669) -> (w1674:dbl[][])  [unwired: 1 in]
                    }
                    n608 = Bundle(cluster=w1660, w1651, w1656) -> (w1661:T14)  [unwired: 9 out]
                  }
                  frame #6 {
                    n609 = property on="Programming scanner" class="Schieberegler (strikt)"("Caption.Text"="") -> ()  [unwired: 2 in, 2 out]
                    n610 = property on="Programming scanner" class="Schieberegler (strikt)"("Val(Sgnl)"=u8 0 ("Wert (signalisierend)")) -> ()  [unwired: 2 in, 2 out]
                  }
                }
                n611 = Unbundle(w1533) -> (w1512:i32[][], "Boolean array"=w1535:bool[])  [unwired: 9 out]
                n612 = case shown="True" "Normalize\nPicture Image" {
                  tunnel: w1512 -> [w1540 w1542]
                  tunnel: [w1540 w1543] -> w1511
                  frame #0 {
                  }
                  frame #1 {
                    n613 = Array Size(array=w1542) -> (size(s)=w1547:i32[])
                    n614 = Array Max & Min(array=w1542) -> (min value=w1541:i32)  [unwired: 3 out]
                    n615 = Index Array(array=w1547, index=0) -> (element=w1545:i32)
                    n616 = Index Array(array=w1547, index=1) -> (element=w1546:i32)
                    n617 = Initialize Array(w1541, w1545, w1546) -> (w1544:i32[][])
                    n618 = Subtract(x=w1542, y=w1544) -> (x-y=w1543:i32[][])
                  }
                }
                n619 = Array Size(array=w1511) -> (size(s)=w1525:i32[])
                n620 = call "Picture_switch_value.vi"("Boolean array in"=w1535, "Value to switch"=7, "Switch"=TRUE) -> ("Boolean array out"=w1532:bool[], "New Value"=w1530:bool)  [unwired: 7 out]
                n621 = Index Array(array=w1525, index=0 ("Index")) -> (element=w1520:i32)
                n622 = Initialize Array(0 ("Element"), w1520, 3 ("Dimension")) -> (w1523:i32[][])
                n623 = property class="Boolesch (strikt)"("Val(Sgnl)"=w1530) -> ()  [unwired: 2 in, 2 out]
                n624 = Replace Array Subset(array=w1511, new element=w1523, index (row)=w1522, index (col)=w1522) -> (w1519:i32[][])
                n625 = Bundle(cluster=w1533, w1519, "Boolean array"=w1532) -> (w1531:T14)  [unwired: 9 out]
              }
            }
            n626 = property on="actual scan stage position" class="Arr (strict)"("Val(Sgnl)"=w1497) -> ()  [unwired: 2 in, 2 out]
          }
          frame #1 {
          }
        }
        n627 = case shown="False" "Overview" {
          tunnel: [w1715 w1721] -> w1305
          tunnel: w1315 -> [w1715 w1719]
          frame #0 {
          }
          frame #1 {
            w1716 = 0.0 ("element")
            w1730 = u16 512 ("Value (Signaling)")
            w1731 = 200.0 ("Value (Signaling)")
            n628 = property class="DigNum (strict)"("Val(Sgnl)"=w1731) -> ()  [unwired: 2 in, 2 out]
            n629 = property on="x-Position" class="DigNum (strict)"("Val(Sgnl)"=w1716) -> ()  [unwired: 2 in, 2 out]
            n630 = property on="z-Position" class="DigNum (strict)"("Val(Sgnl)"=w1716) -> ()  [unwired: 2 in, 2 out]
            n631 = property on="y-Position" class="DigNum (strict)"("Val(Sgnl)"=w1716) -> ()  [unwired: 2 in, 2 out]
            n632 = property on="x-Pixel" class="DigNum (strict)"("Val(Sgnl)"=w1730) -> ()  [unwired: 2 in, 2 out]
            n633 = property on="y-Pixel" class="DigNum (strict)"("Val(Sgnl)"=w1730) -> ()  [unwired: 2 in, 2 out]
            n634 = Build Array(0.0 ("y"), 200.0 ("y")) -> (w1724:dbl[])
            n635 = Build Array(0.0 ("y"), 200.0 ("y")) -> (w1723:dbl[])
            n636 = Build Array(200.0 ("y")) -> (w1722:dbl[])
            n637 = Build Array(w1724, w1723, w1722) -> (w1720:dbl[][])
            n638 = Build Array "Scanner position"(w1716, w1716, w1716) -> (w1718:dbl[])
            n639 = property on="Picture size" class="DigNum (strict)"("Val(Sgnl)"=w1731) -> ()  [unwired: 2 in, 2 out]
            n640 = Bundle "Scanner pos"(w1718, w1718) -> (w1717:cluster{dbl[], dbl[]})  [unwired: 1 out]
            n641 = Bundle(cluster=w1719, w1720, w1717) -> (w1721:T14)  [unwired: 9 out]
          }
        }
        n642 = call "Picture_View_ROI.vi"("Input Cluster"=w1305, "ROI"="ROI", "Cluster 2"=w1308) -> ("ROI-Picture"=w1311:i32[][], "Out of range"=w1312:bool[])  [unwired: 1 in, 6 out]
        n643 = case shown="True" "Zoom" {
          tunnel: w1308 -> [_ w1411]
          tunnel: w1305 -> [w1401 w1410]
          tunnel: [w1401 w1408] -> w1309
          frame #0 {
          }
          frame #1 {
            n644 = call "ROI_Picture_size.vi"("Input Cluster"=w1410, "Pixel"=w1411) -> ("output cluster"=w1408:T14)  [unwired: 1 in, 8 out]
            n645 = property on="ROI" class="Bool (strict)"("Val(Sgnl)"=FALSE ("Value (Signaling)")) -> ()  [unwired: 2 in, 2 out]
            n646 = Unbundle(w1408) -> ("cluster"=w1407:T6)  [unwired: 10 out]
            n647 = Unbundle(w1407) -> ("x-Position"=w1404:dbl, "y-Position"=w1405:dbl, "Picture size"=w1402:dbl, w1403:dbl, "z-Position"=w1406:dbl)  [unwired: 3 out]
            n648 = property on="x-Position" class="DigNum (strict)"("Val(Sgnl)"=w1404) -> ()  [unwired: 2 in, 2 out]
            n649 = property on="y-Position" class="DigNum (strict)"("Val(Sgnl)"=w1405) -> ()  [unwired: 2 in, 2 out]
            n650 = property class="DigNum (strict)"("Val(Sgnl)"=w1403) -> ()  [unwired: 2 in, 2 out]
            n651 = property on="z-Position" class="DigNum (strict)"("Val(Sgnl)"=w1406) -> ()  [unwired: 2 in, 2 out]
            n652 = property on="Picture size" class="DigNum (strict)"("Val(Sgnl)"=w1402) -> ()  [unwired: 2 in, 2 out]
          }
        }
        n653 = call "Picture_shr_Save_to_matlab.vi"("Input Cluster"=w1305, "Stack"=w1294, "Mode"="?", "Save"="Save") -> ()  [unwired: 8 out]
        n654 = Boolean Array To Number(Boolean array=w1312) -> (number=w1314:u32)
        n655 = Not Equal To 0?(x=w1314) -> (x != 0?=w1313:bool)
        n656 = case shown="True" w1313 {
          tunnel: w1312 -> [_ w1419]
          tunnel: w1311 -> [_ w1417]
          frame #0 {
          }
          frame #1 {
            n657 = Array Size(array=w1417) -> (size(s)=w1416:i32[])
            n658 = Index Array(array=w1416, index=0) -> (element=w1412:i32)
            n659 = Index Array(array=w1416, index=1) -> (element=w1413:i32)
            n660 = for {
              N: 4 -> [_]
              tunnel: w1419 -> [w1422] mode=indexing
              tunnel: w1413 -> [w1421]
              tunnel: w1412 -> [w1420]
              i -> [w1423]
              n661 = case shown="3" w1423 {
                tunnel: w1422 -> [_ _ _ _]
                tunnel: w1421 -> [_ _ w1434 w1438]
                tunnel: w1420 -> [w1427 w1431 _ _]
                frame #0 {
                  n662 = Multiply(x=w1427, y=0.1 ("Value (Signaling)")) -> (x*y=w1425:dbl)
                  n663 = To Long Integer(number=w1425) -> (32bit integer=w1424:i32)
                  n664 = property on="left limit" class="DigNum (strict)"("Val(Sgnl)"=w1424) -> ()  [unwired: 2 in, 2 out]
                }
                frame #1 {
                  n665 = Multiply(x=w1431, y=0.2 ("Value (Signaling)")) -> (x*y=w1430:dbl)
                  n666 = Subtract(x=w1431, y=w1430) -> (x-y=w1429:dbl)
                  n667 = To Long Integer(number=w1429) -> (32bit integer=w1428:i32)
                  n668 = property on="x-Pixel" class="DigNum (strict)"("Val(Sgnl)"=w1428) -> ()  [unwired: 2 in, 2 out]
                }
                frame #2 {
                  n669 = Multiply(x=w1434, y=0.1 ("Value (Signaling)")) -> (x*y=w1435:dbl)
                  n670 = To Long Integer(number=w1435) -> (32bit integer=w1433:i32)
                  n671 = property on="lower limit" class="DigNum (strict)"("Val(Sgnl)"=w1433) -> ()  [unwired: 2 in, 2 out]
                }
                frame #3 {
                  n672 = Multiply(x=w1438, y=0.2 ("Value (Signaling)")) -> (x*y=w1440:dbl)
                  n673 = Subtract(x=w1438, y=w1440) -> (x-y=w1439:dbl)
                  n674 = To Long Integer(number=w1439) -> (32bit integer=w1437:i32)
                  n675 = property on="y-Pixel" class="DigNum (strict)"("Val(Sgnl)"=w1437) -> ()  [unwired: 2 in, 2 out]
                }
              }
            }
          }
        }
        "?" <- "ROI"
      }
    }
    "Intensity Graph" <- w1096
    n676 = property class="TabCtl (strict)"() -> ("Value"=w1093:T1)  [unwired: 2 in, 2 out]
    n677 = property class="DigNum (strict)"("Visible"=w1114) -> ()  [unwired: 2 in, 2 out]
    n678 = property class="DigNum (strict)"("Visible"=w1114) -> ()  [unwired: 2 in, 2 out]
    n679 = flat-sequence {
      tunnel: w1107 -> [w1132]
      tunnel: [w1130] -> w1095
      tunnel: [w1142] -> w1101
      tunnel: w1095 -> [w1142]
      tunnel: [w1140] -> _
      frame #0 {
        n680 = Unbundle(w1132) -> ("Boolean array"=w1133:bool[])  [unwired: 10 out]
        n681 = call "Andor_iXon_Cooling.vi"("Boolean array in"=w1133, "target temperature / [°C]"="target temperature / [°C]", "Cooling"="Cooling") -> ("Boolean array out"=w1131:bool[])  [unwired: 8 out]
        n682 = Bundle(cluster=w1132, "Boolean array"=w1131) -> (w1130:T14)  [unwired: 10 out]
        n683 = Index Array(array=w1131, index=1) -> (element=→"On/Off":bool)
      }
      frame #1 {
        n684 = call "SetEMGainMode.vi"("mode"="mode") -> ("error out"=w1141:errorcluster)  [unwired: 1 in, 1 out]
        n685 = call "SetEMCCDGain.vi"("error in (no error)"=w1141, "gain"="gain") -> ("error out"=w1140:errorcluster)  [unwired: 1 out]
      }
    }
    n686 = Not(x=w1114) -> (.not. x?=w1115:bool)
    n687 = property on="Intensity Graph" class="IntGraph (strict)"("Visible"=w1114) -> ()  [unwired: 2 in, 2 out]
    n688 = property on="Intensity Graph" class="IntGraph (strict)"("Cursor.Visible"=w1113) -> ()  [unwired: 2 in, 2 out]
    n689 = case shown="\"Alignment\"" w1093 {
      tunnel: w1096 -> [_ _ _ _ _ _ _ w1118 _]
      frame #0 {
      }
      frame #1 {
      }
      frame #2 {
      }
      frame #3 {
      }
      frame #4 {
      }
      frame #5 {
      }
      frame #6 {
      }
      frame #7 {
        n690 = script code="[x,y] = meshgrid(1:size(Data,2),1:size(Data,1));\nx1 = sum(sum(x.*Data))/sum(sum(Data));\nx2 = sum(sum(x.^2.*Data))/sum(sum(Data));\ny1 = sum(sum(y.*Data))/sum(sum(Data));\ny2 = sum(sum(y.^2.*Data))/sum(sum(Data));\nsigx = sqrt(x2-x1^2);\nsigy = sqrt(y2-y1^2);"("Data"=w1118) -> ("sigx"=w1121:dbl, "sigy"=w1119:dbl)  [unwired: 2 out]
        "sigx" <- w1121
        "sigy" <- w1119
        n691 = Bundle(w1121, w1119) -> (→"Signalverlaufsdiagramm":cluster{dbl, dbl})  [unwired: 1 out]
      }
      frame #8 {
      }
    }
    n692 = property on="Waveform Chart 2" class="WFChart (strict)"("Visible"=w1115) -> ()  [unwired: 2 in, 2 out]
    n693 = case shown="True" "Shut down\ncamera" {
      tunnel: [errorcluster {"status"=FALSE, "code"=0, "source"=""} ("error out") w1123] -> _
      frame #0 {
      }
      frame #1 {
        n694 = call "ShutDown.vi"() -> ("error out"=w1123:errorcluster)  [unwired: 2 in, 1 out]
      }
    }
    n695 = flat-sequence {
      tunnel: w1101 -> [w1129]
      tunnel: [w1128] -> w1100
      frame #0 {
        n696 = Unbundle(w1129) -> (w1127:T13)  [unwired: 10 out]
        n697 = Bundle(cluster=w1127, "Horizontal bin"="x-pixels", "Vertical bin"="y-pixels") -> (w1126:T13)  [unwired: 14 out]
        n698 = Bundle(cluster=w1129, w1126) -> (w1128:T14)  [unwired: 10 out]
      }
    }
    n699 = Unbundle(w1101) -> ("Boolean array"=w1106:bool[])  [unwired: 10 out]
    n700 = Index Array(array=w1106, index=7) -> (element=w1109:bool)
    n701 = case shown="False" w1109 {
      tunnel: w1100 -> [w1177 w1195]
      tunnel: [w1178 w1195] -> w1105
      frame #0 {
        n702 = Unbundle(w1177) -> ("Boolean array"=w1176:bool[])  [unwired: 10 out]
        n703 = Index Array(array=w1176, index=0) -> (element=w1179:bool)
        n704 = case shown="False" w1179 {
          tunnel: [w1185 w1190] -> _
          tunnel: w1177 -> [w1183 w1189]
          tunnel: [w1181 w1189] -> w1178
          frame #0 {
            n705 = Unbundle(w1183) -> (w1188:T13, "Boolean array"=w1184:bool[])  [unwired: 9 out]
            n706 = call "Andor_iXon_Init.vi"("input cluster"=w1188) -> ("error out"=w1185:errorcluster)  [unwired: 1 in, 9 out]
            n707 = Replace Array Subset(array=w1184, new element=TRUE ("new element/subarray"), index=0) -> (w1182:bool[])
            n708 = Bundle(cluster=w1183, "Boolean array"=w1182) -> (w1181:T14)  [unwired: 10 out]
          }
          frame #1 {
            w1193 = 36  # DRV_TEMP_STABILIZED
            n709 = call "GetTemperature.vi"() -> ("error out"=w1190:errorcluster, "status"=w1194:T27, "temperature"=→"act. temperature / [°C]":i32)  [unwired: 1 in, 4 out]
            n710 = Equal?(x=w1194, y=w1193) -> (x = y?=→"Temp-stabilized":bool)
          }
        }
      }
      frame #1 {
      }
    }
    n711 = property on="stop" class="Bool (strict)"() -> ("Value"=w1117:bool)  [unwired: 2 in, 2 out]
  }
  n712 = call <vilib>:"DAQmx Clear Task.vi"("task in"=w10, "error in"=w11) -> ()  [unwired: 14 out]
  n713 = VISA Close(VISA resource name=w44, error in (no error)=w43) -> ()  [unwired: 1 out]
  n714 = call <vilib>:"DAQmx Stop Task.vi"("task/channels in"=w25, "error in"=w24) -> ("task out"=w27:refnum<k21>, "error out"=w26:errorcluster)  [unwired: 12 out]
  n715 = call <vilib>:"DAQmx Clear Task.vi"("task in"=w27, "error in"=w26) -> ()  [unwired: 14 out]
